vi "GOLPI Config Panel.vi"(8 "error in":errorcluster, 11 "session in":T2={"adc"={"niScope"={"channel cfg"=[], "sessions"=[], "multi cards"=FALSE, "channels"=0, "type"=enum."n/a", "memory [B/chn]"=0, "ext. clock [Hz]"=0.0, "samples count"=0, "use streaming"=FALSE, "proc setup"={"packet size [smpl]"=0, "current timeout [s]"=0.0, "blk2blk timeout [s]"=0.0, "event time"=timestamp(0 s since 1904-01-01), "temp sampl T [s]"=0.0, "data queue"=refnum, "stop notifier"=refnum, "proc ref"=refnum}, "sample width [B]"=0, "ranges [V]"=[], "trigger setup"={"coupling"=1, "level [V]"=0.0, "slope"=0, "mode"=enum."Immediate", "pre-trigger [%]"=0.0}, "fs [Hz]"=0.0, "bitres [bit]"=0, "clock source"=enum."VAL_NO_SOURCE"}, "3458A"={"channels"=[], "sync unit"={"VISA"="", "type"=enum."Picotest U6200A"}, "awg unit"={"type"=enum."Agilent 331xxA to 332xxA", "VISA"="", "enable 10MHz ref"=FALSE, "cmi ckd2"={"VISA"="", "clock source"=enum."Auto", "manual ref clk"=FALSE, "ref clock [Hz]"=0.0, "div mode"=enum."Set divisor directly"}, "cmi sync v3"={"VISA"="", "baud rate [bd/s]"=115200, "source"=enum."Auto", "hv range"=enum."1kV", "fsrc is fixed"=FALSE, "fsrc [Hz]"=10000000.0, "freq integ [s]"=1.0, "freq filter"=5, "trig level"=enum."TTL 5V", "chn1 mode"=enum."Source divider", "chn1 level"=enum."Positive 5V", "chn2 mode"=enum."Source divider", "chn2 level"=enum."Positive 5V", "chn2 div"=1, "chn3 mode"=enum."Chn 1 Active", "chn3 level"=enum."Positive 5V", "chn1 div entry"=enum."Calculate nearest divisor from measured fx", "chn1 dev limit [%]"=1.0, "chn1 check dev"=FALSE}, "trigger"={"source"=enum."Immediate", "slope"=enum."POS", "coupling"=enum."DC", "level [V]"=0.0, "hysteresis [V]"=0.0, "pre-trigger [%]"=0.0}, "HMF2500 cfg"={"Baud Rate"=9600, "Parity"=0, "Data Bits"=8, "Flow Control"=4}}, "sync mode"=enum."MASTER-SLAVE, MASTER clocked by TIMER", "streaming mode"=FALSE, "idn mode"=enum."Auto", "sampling mode"=enum."DCV", "sample memory [B]"=0, "proc setup"={"channel id"=0, "packet size [smpl]"=0, "current timeout [s]"=0.0, "blk2blk timeout [s]"=0.0, "event time"=timestamp(0 s since 1904-01-01), "stop notifier"=refnum, "data queues"=[], "proc refs"=[], "bus semaphore"=refnum}, "sample size [B]"=0, "sample count"=0, "aux data"={"channel id"=0, "valid?"=[], "gain [V]"=[], "timestamp [s]"=[], "Ts [s]"=0.0, "abs timestamp"=timestamp(0 s since 1904-01-01), "t [deg C]"=[], "multiplex timestamp [s]"=-1.0, "only multiplex?"=FALSE, "multiplex smpl offset"=0, "overflow?"=FALSE}, "ranges [V]"=[], "aperture [s]"=0.0, "LEVEL trigger"={"edge"=enum."POS", "level [V]"=0.0, "coupling"=enum."DC"}, "trigger mode"=enum."AUTO", "measure temp.?"=FALSE, "disp mesages"=[], "shared bus?"=FALSE, "disable display?"=FALSE, "aper mode"=enum."Manual", "aper rules"=[], "multiplex"={"cycles"=0, "delay [s]"=0.0, "enabled"=FALSE, "overhead [s]"=1.0, "tot smpls"=0, "sub-rec"=0, "overhead [%]"=0.0, "emulated"=FALSE}, "F8588 lpf"=enum."Off", "F8588 pll"=enum."Off", "F8588 couple"=enum."DC, auto", "fs"={"freq mode"=enum."fs or Ts", "fs [Hz]"=0.0, "fref [Hz]"=0.0, "mul"=0.0, "div"=0.0}, "fs mode"=enum."fs or Ts", "init timestamp"=timestamp(0 s since 1904-01-01), "last report timestamp"=timestamp(0 s since 1904-01-01)}, "dsdll"={"dsdll"={"dsdll path"=path "", "dsdll handle"=[], "output devices"=[], "capture devices"=[]}, "channels"=0, "device id"=0, "channel idns"=[], "proc setup"={"packet size [smpl]"=0, "current timeout [s]"=0.0, "blk2blk timeout [s]"=0.0, "event time"=timestamp(0 s since 1904-01-01), "data queue"=refnum, "stop notifier"=refnum, "proc ref"=refnum}, "samples count"=0, "fs [Hz]"=0.0}, "type"=enum."niScope", "channel idn str"=[], "aux instr idn str"=[], "modified?"=FALSE, "simadc"={"channels"=[], "range [V]"=0.0, "Ts step [s]"=0.0, "time [s]"=0.0, "fs [Hz]"=0.0, "count"=0, "smpl offset"=0, "set count"=0, "bit res"=0}, "force rst?"=FALSE, "exit mode"=enum."Immediate reset", "exit dly"=0.0, "exit tmr"=timestamp(0 s since 1904-01-01), "busy?"=FALSE, "accessed?"=FALSE, "multiplex"={"Type"=enum."Dummy", "gen com ssn"={"visa"="", "primary"=enum."None", "secondary"=enum."None", "channels"=[]}, "delay before [s]"=0.0, "delay post [s]"=0.0, "sequence"=[], "enabled"=FALSE, "ref timestamp [s]"=0.0, "idn string"="", "dev niScope"="", "niScope idx"=0, "QPMX ssn"={"visa"="", "switch mode"=enum."Switched by TWM", "sequence"=[], "timing delays"=[], "polarity"=enum."Positive", "ss delay (s)"=2.0, "internal timer (s)"=1.0, "Last loaded sequence file"=path "", "startup delay (s)"=2.0}, "VISA mux ssn"={"VISA"="", "paths"=[], "idn command"="", "serial cfg"={"Baud rate"=9600, "Data bits"=8, "Parity"=0, "Stop bits"=10, "Flow control"=0, "End Mode Read"=enum."None", "End Mode Write"=enum."None", "Term character"=0, "Term enable"=FALSE}}}, "keysight dso"={"VISA"="", "channels"=[], "bw limit [Hz]"=0.0, "resolution"=enum."Basic", "trig noise reject"=enum."Normal", "N"=0, "trigger config"={"trigger source"=enum."Immediate", "trigger slope"=enum."Negative", "level [V]"=0.0, "hysteresis [V]"=0.001, "pre-trig [%]"=50}, "fs [Hz]"=0.0, "timeout stop"=timestamp(0 s since 1904-01-01), "waiting for opc"=FALSE, "fetch offset [smpl]"=0, "abs timestamp"=timestamp(0 s since 1904-01-01), "ranges [V]"=[], "decimation"=1.0, "ext ref"=FALSE, "emulate aperture"=FALSE, "model"=enum."DSO91304"}, "cdaq"={"mclk [Hz]"=12800000.0, "ADC task"="", "mclk reference"="", "fs [Hz]"=50000.0, "queue adc cmd"=refnum, "queue adc data"=refnum, "adc proc ref"=refnum, "channels"=[], "last channels"=[], "timeout"=timestamp(0 s since 1904-01-01), "N"=1000, "mclk mode"=enum."Free running", "ext mclk source"=""}, "ignore overload"=FALSE, "ADS127L21"={"VISA"="", "chn list"=[], "record size"=0, "phys. channels"=0, "adc fifo size"=0, "channels"=[], "ext refclk?"=FALSE, "fs [Hz]"=0.0, "ext refclk [Hz]"=0.0, "meas refclk [Hz]"=0.0, "EXTOUT mode"=enum."ADCCLK", "EXTOUT polarity"=enum."NORM", "EXTOUT divisor"=0}}, "sequence"=[], "sequence setup"={"group setups"=[], "rec count"=0, "range mode"=enum."Keep defaults", "fs mode"=enum."Frequency", "rng even"=0.0, "rng odd"=0.0, "folder"=path "", "name base"="", "meas id"=0, "settle [s]"=0.0, "comment"="", "avg count"=0, "fs-abs-fr fr"=0.0, "fs-abs-fr fs"=0.0, "fs-div fr"=0.0, "fs-div div"=0.0, "fs-mn fr"=0.0, "fs-mn mul"=0.0, "fs-mn div"=0.0, "fs-rat fr"=0.0, "fs-rat rat"=0.0}, "golpi"=refnum, "processing setup"={"mode"=enum."Raw", "call after avgs?"=FALSE, "calculate?"=FALSE, "raw mode"={"command"="", "result mode"=enum."Display console output (only Octave)", "res variable"=""}, "QWTB"={"QWTB path"=path "", "alg filter path"="", "alg ids"=[], "alg parameters"=[], "parsed parameters"=[], "selected alg id"="", "selected unc mode"=enum."None", "qwtb mcc"=100, "qwtb timeout"=90, "qwtb covg"=95.0, "qwtb ofs"=0, "qwtb lim data"=0, "multicore"={"jobs folder"=path "", "cores"=0, "max jobs"=0, "mode"=enum."Singlecore"}, "unc once?"=FALSE, "qwtb tstemp"=enum."Enabled (default)", "octave reset"=FALSE, "exec mode"=enum."Single-core"}}, "corrections"={"transducers"={"channels"=[], "last path"=path "", "root path"=path ""}, "digitizer"={"last path"=path "", "channel paths"=[], "channel idns"=[], "correction name"="", "channel names"=[], "folders to copy"=[], "channel valid"=[], "correction path"=path "", "correction rel path"="", "rel folders to copy"=[], "root path"=path ""}}, "assist cfg"={"P"=0, "Q"=0, "rel shift"=0.0, "ref freq"=0.0, "min fs"=0.0, "max fs tol"=0.0, "min int"=0.0, "max int"=0.0, "max err"=0.0, "max timeout"=0.0}} {"corrections"."transducers"."channels"."Phase index" min=1 step=1; "adc"."ADS127L21"."channels"."Channel" min=1 max=8 step=1; "adc"."ADS127L21"."channels"."Range [Vpk]" items=["±1.65V", "±2V"]; "adc"."cdaq"."last channels"."Channel id" min=0 step=1; "adc"."cdaq"."channels"."Channel id" min=0 step=1; "adc"."keysight dso"."decimation" min=1.0; "adc"."keysight dso"."bw limit [Hz]" format="%#_6p"; "adc"."keysight dso"."channels"."Offset [V]" format="%#_6p"; "adc"."keysight dso"."channels"."Range [Vpk]" min=0.0 format="%#_6p"; "adc"."keysight dso"."channels"."Channel" min=1; "adc"."multiplex"."VISA mux ssn"."serial cfg"."Flow control" items=["None", "XON/XOFF", "CTS/RTS", "XON/XOFF + CTS/RTS", "DTR/DSR", "XON/XOFF + DTR/DSR"]; "adc"."multiplex"."VISA mux ssn"."serial cfg"."Stop bits" items=["1 bit"=10, "1.5 bits"=15, "2 bits"=20]; "adc"."multiplex"."VISA mux ssn"."serial cfg"."Parity" items=["None", "Odd", "Even", "Mark", "Space"]; "adc"."multiplex"."VISA mux ssn"."serial cfg"."Data bits" items=["5 bits"=5, "6 bits"=6, "7 bits"=7, "8 bits"=8]; "adc"."multiplex"."VISA mux ssn"."serial cfg"."Baud rate" items=["150 Bd"=150, "300 Bd"=300, "600 Bd"=600, "1200 Bd"=1200, "2400 Bd"=2400, "4800 Bd"=4800, "9600 Bd"=9600, "19.2 kBd"=19200, "38.4 kBd"=38400, "57.6 kBd"=57600, "115.2 kBd"=115200]; "adc"."multiplex"."QPMX ssn"."startup delay (s)" min=0.0 step=1.0; "adc"."multiplex"."QPMX ssn"."internal timer (s)" min=0.0 step=1.0; "adc"."multiplex"."QPMX ssn"."ss delay (s)" min=0.0 step=1.0; "adc"."multiplex"."QPMX ssn"."timing delays" min=1 max=255 step=1; "adc"."3458A"."awg unit"."HMF2500 cfg"."Flow Control" items=["None", "XON/XOFF", "RTS/CTS", "XON/XOFF & RTS/CTS", "DTR/DSR", "XON/XOFF & DTR/DSR"]; "adc"."3458A"."awg unit"."HMF2500 cfg"."Data Bits" items=["7"=7, "8"=8]; "adc"."3458A"."awg unit"."HMF2500 cfg"."Parity" items=["None", "Odd", "Even", "Mark", "Space"]; "adc"."3458A"."awg unit"."HMF2500 cfg"."Baud Rate" items=["300"=300, "600"=600, "1200"=1200, "2400"=2400, "4800"=4800, "9600"=9600, "19200"=19200]; "adc"."3458A"."awg unit"."cmi sync v3"."chn2 div" min=1 max=100000000 step=1; "adc"."3458A"."awg unit"."cmi sync v3"."fsrc [Hz]" format="%_8p"; "adc"."3458A"."channels"."Range [Vpk]" min=0.0; "adc"."niScope"."trigger setup"."pre-trigger [%]" format="%.2f"; "adc"."niScope"."trigger setup"."level [V]" format="%.2f"; "adc"."niScope"."trigger setup"."coupling" items=["AC"=0, "DC"=1, "HF Reject"=3, "LF Reject"=4, "AC Plus HF Reject"=1001]; "adc"."niScope"."channel cfg"."Range [Vpk]" min=0.0; "adc"."niScope"."channel cfg"."Channel" min=0}) -> (0 "error out":errorcluster, 3 "session out":T2={"adc"={"niScope"={"channel cfg"=[], "sessions"=[], "multi cards"=FALSE, "channels"=0, "type"=enum."n/a", "memory [B/chn]"=0, "ext. clock [Hz]"=0.0, "samples count"=0, "use streaming"=FALSE, "proc setup"={"packet size [smpl]"=0, "current timeout [s]"=0.0, "blk2blk timeout [s]"=0.0, "event time"=timestamp(0 s since 1904-01-01), "temp sampl T [s]"=0.0, "data queue"=refnum, "stop notifier"=refnum, "proc ref"=refnum}, "sample width [B]"=0, "ranges [V]"=[], "trigger setup"={"coupling"=1, "level [V]"=0.0, "slope"=0, "mode"=enum."Immediate", "pre-trigger [%]"=0.0}, "fs [Hz]"=0.0, "bitres [bit]"=0, "clock source"=enum."VAL_NO_SOURCE"}, "3458A"={"channels"=[], "sync unit"={"VISA"="", "type"=enum."Picotest U6200A"}, "awg unit"={"type"=enum."Agilent 331xxA to 332xxA", "VISA"="", "enable 10MHz ref"=FALSE, "cmi ckd2"={"VISA"="", "clock source"=enum."Auto", "manual ref clk"=FALSE, "ref clock [Hz]"=0.0, "div mode"=enum."Set divisor directly"}, "cmi sync v3"={"VISA"="", "baud rate [bd/s]"=115200, "source"=enum."Auto", "hv range"=enum."1kV", "fsrc is fixed"=FALSE, "fsrc [Hz]"=10000000.0, "freq integ [s]"=1.0, "freq filter"=5, "trig level"=enum."TTL 5V", "chn1 mode"=enum."Source divider", "chn1 level"=enum."Positive 5V", "chn2 mode"=enum."Source divider", "chn2 level"=enum."Positive 5V", "chn2 div"=1, "chn3 mode"=enum."Chn 1 Active", "chn3 level"=enum."Positive 5V", "chn1 div entry"=enum."Calculate nearest divisor from measured fx", "chn1 dev limit [%]"=1.0, "chn1 check dev"=FALSE}, "trigger"={"source"=enum."Immediate", "slope"=enum."POS", "coupling"=enum."DC", "level [V]"=0.0, "hysteresis [V]"=0.0, "pre-trigger [%]"=0.0}, "HMF2500 cfg"={"Baud Rate"=9600, "Parity"=0, "Data Bits"=8, "Flow Control"=4}}, "sync mode"=enum."MASTER-SLAVE, MASTER clocked by TIMER", "streaming mode"=FALSE, "idn mode"=enum."Auto", "sampling mode"=enum."DCV", "sample memory [B]"=0, "proc setup"={"channel id"=0, "packet size [smpl]"=0, "current timeout [s]"=0.0, "blk2blk timeout [s]"=0.0, "event time"=timestamp(0 s since 1904-01-01), "stop notifier"=refnum, "data queues"=[], "proc refs"=[], "bus semaphore"=refnum}, "sample size [B]"=0, "sample count"=0, "aux data"={"channel id"=0, "valid?"=[], "gain [V]"=[], "timestamp [s]"=[], "Ts [s]"=0.0, "abs timestamp"=timestamp(0 s since 1904-01-01), "t [deg C]"=[], "multiplex timestamp [s]"=-1.0, "only multiplex?"=FALSE, "multiplex smpl offset"=0, "overflow?"=FALSE}, "ranges [V]"=[], "aperture [s]"=0.0, "LEVEL trigger"={"edge"=enum."POS", "level [V]"=0.0, "coupling"=enum."DC"}, "trigger mode"=enum."AUTO", "measure temp.?"=FALSE, "disp mesages"=[], "shared bus?"=FALSE, "disable display?"=FALSE, "aper mode"=enum."Manual", "aper rules"=[], "multiplex"={"cycles"=0, "delay [s]"=0.0, "enabled"=FALSE, "overhead [s]"=1.0, "tot smpls"=0, "sub-rec"=0, "overhead [%]"=0.0, "emulated"=FALSE}, "F8588 lpf"=enum."Off", "F8588 pll"=enum."Off", "F8588 couple"=enum."DC, auto", "fs"={"freq mode"=enum."fs or Ts", "fs [Hz]"=0.0, "fref [Hz]"=0.0, "mul"=0.0, "div"=0.0}, "fs mode"=enum."fs or Ts", "init timestamp"=timestamp(0 s since 1904-01-01), "last report timestamp"=timestamp(0 s since 1904-01-01)}, "dsdll"={"dsdll"={"dsdll path"=path "", "dsdll handle"=[], "output devices"=[], "capture devices"=[]}, "channels"=0, "device id"=0, "channel idns"=[], "proc setup"={"packet size [smpl]"=0, "current timeout [s]"=0.0, "blk2blk timeout [s]"=0.0, "event time"=timestamp(0 s since 1904-01-01), "data queue"=refnum, "stop notifier"=refnum, "proc ref"=refnum}, "samples count"=0, "fs [Hz]"=0.0}, "type"=enum."niScope", "channel idn str"=[], "aux instr idn str"=[], "modified?"=FALSE, "simadc"={"channels"=[], "range [V]"=0.0, "Ts step [s]"=0.0, "time [s]"=0.0, "fs [Hz]"=0.0, "count"=0, "smpl offset"=0, "set count"=0, "bit res"=0}, "force rst?"=FALSE, "exit mode"=enum."Immediate reset", "exit dly"=0.0, "exit tmr"=timestamp(0 s since 1904-01-01), "busy?"=FALSE, "accessed?"=FALSE, "multiplex"={"Type"=enum."Dummy", "gen com ssn"={"visa"="", "primary"=enum."None", "secondary"=enum."None", "channels"=[]}, "delay before [s]"=0.0, "delay post [s]"=0.0, "sequence"=[], "enabled"=FALSE, "ref timestamp [s]"=0.0, "idn string"="", "dev niScope"="", "niScope idx"=0, "QPMX ssn"={"visa"="", "switch mode"=enum."Switched by TWM", "sequence"=[], "timing delays"=[], "polarity"=enum."Positive", "ss delay (s)"=2.0, "internal timer (s)"=1.0, "Last loaded sequence file"=path "", "startup delay (s)"=2.0}, "VISA mux ssn"={"VISA"="", "paths"=[], "idn command"="", "serial cfg"={"Baud rate"=9600, "Data bits"=8, "Parity"=0, "Stop bits"=10, "Flow control"=0, "End Mode Read"=enum."None", "End Mode Write"=enum."None", "Term character"=0, "Term enable"=FALSE}}}, "keysight dso"={"VISA"="", "channels"=[], "bw limit [Hz]"=0.0, "resolution"=enum."Basic", "trig noise reject"=enum."Normal", "N"=0, "trigger config"={"trigger source"=enum."Immediate", "trigger slope"=enum."Negative", "level [V]"=0.0, "hysteresis [V]"=0.001, "pre-trig [%]"=50}, "fs [Hz]"=0.0, "timeout stop"=timestamp(0 s since 1904-01-01), "waiting for opc"=FALSE, "fetch offset [smpl]"=0, "abs timestamp"=timestamp(0 s since 1904-01-01), "ranges [V]"=[], "decimation"=1.0, "ext ref"=FALSE, "emulate aperture"=FALSE, "model"=enum."DSO91304"}, "cdaq"={"mclk [Hz]"=12800000.0, "ADC task"="", "mclk reference"="", "fs [Hz]"=50000.0, "queue adc cmd"=refnum, "queue adc data"=refnum, "adc proc ref"=refnum, "channels"=[], "last channels"=[], "timeout"=timestamp(0 s since 1904-01-01), "N"=1000, "mclk mode"=enum."Free running", "ext mclk source"=""}, "ignore overload"=FALSE, "ADS127L21"={"VISA"="", "chn list"=[], "record size"=0, "phys. channels"=0, "adc fifo size"=0, "channels"=[], "ext refclk?"=FALSE, "fs [Hz]"=0.0, "ext refclk [Hz]"=0.0, "meas refclk [Hz]"=0.0, "EXTOUT mode"=enum."ADCCLK", "EXTOUT polarity"=enum."NORM", "EXTOUT divisor"=0}}, "sequence"=[], "sequence setup"={"group setups"=[], "rec count"=0, "range mode"=enum."Keep defaults", "fs mode"=enum."Frequency", "rng even"=0.0, "rng odd"=0.0, "folder"=path "", "name base"="", "meas id"=0, "settle [s]"=0.0, "comment"="", "avg count"=0, "fs-abs-fr fr"=0.0, "fs-abs-fr fs"=0.0, "fs-div fr"=0.0, "fs-div div"=0.0, "fs-mn fr"=0.0, "fs-mn mul"=0.0, "fs-mn div"=0.0, "fs-rat fr"=0.0, "fs-rat rat"=0.0}, "golpi"=refnum, "processing setup"={"mode"=enum."Raw", "call after avgs?"=FALSE, "calculate?"=FALSE, "raw mode"={"command"="", "result mode"=enum."Display console output (only Octave)", "res variable"=""}, "QWTB"={"QWTB path"=path "", "alg filter path"="", "alg ids"=[], "alg parameters"=[], "parsed parameters"=[], "selected alg id"="", "selected unc mode"=enum."None", "qwtb mcc"=100, "qwtb timeout"=90, "qwtb covg"=95.0, "qwtb ofs"=0, "qwtb lim data"=0, "multicore"={"jobs folder"=path "", "cores"=0, "max jobs"=0, "mode"=enum."Singlecore"}, "unc once?"=FALSE, "qwtb tstemp"=enum."Enabled (default)", "octave reset"=FALSE, "exec mode"=enum."Single-core"}}, "corrections"={"transducers"={"channels"=[], "last path"=path "", "root path"=path ""}, "digitizer"={"last path"=path "", "channel paths"=[], "channel idns"=[], "correction name"="", "channel names"=[], "folders to copy"=[], "channel valid"=[], "correction path"=path "", "correction rel path"="", "rel folders to copy"=[], "root path"=path ""}}, "assist cfg"={"P"=0, "Q"=0, "rel shift"=0.0, "ref freq"=0.0, "min fs"=0.0, "max fs tol"=0.0, "min int"=0.0, "max int"=0.0, "max err"=0.0, "max timeout"=0.0}} {"corrections"."transducers"."channels"."Phase index" min=1 step=1; "adc"."ADS127L21"."channels"."Channel" min=1 max=8 step=1; "adc"."ADS127L21"."channels"."Range [Vpk]" items=["±1.65V", "±2V"]; "adc"."cdaq"."last channels"."Channel id" min=0 step=1; "adc"."cdaq"."channels"."Channel id" min=0 step=1; "adc"."keysight dso"."decimation" min=1.0; "adc"."keysight dso"."bw limit [Hz]" format="%#_6p"; "adc"."keysight dso"."channels"."Offset [V]" format="%#_6p"; "adc"."keysight dso"."channels"."Range [Vpk]" min=0.0 format="%#_6p"; "adc"."keysight dso"."channels"."Channel" min=1; "adc"."multiplex"."VISA mux ssn"."serial cfg"."Flow control" items=["None", "XON/XOFF", "CTS/RTS", "XON/XOFF + CTS/RTS", "DTR/DSR", "XON/XOFF + DTR/DSR"]; "adc"."multiplex"."VISA mux ssn"."serial cfg"."Stop bits" items=["1 bit"=10, "1.5 bits"=15, "2 bits"=20]; "adc"."multiplex"."VISA mux ssn"."serial cfg"."Parity" items=["None", "Odd", "Even", "Mark", "Space"]; "adc"."multiplex"."VISA mux ssn"."serial cfg"."Data bits" items=["5 bits"=5, "6 bits"=6, "7 bits"=7, "8 bits"=8]; "adc"."multiplex"."VISA mux ssn"."serial cfg"."Baud rate" items=["150 Bd"=150, "300 Bd"=300, "600 Bd"=600, "1200 Bd"=1200, "2400 Bd"=2400, "4800 Bd"=4800, "9600 Bd"=9600, "19.2 kBd"=19200, "38.4 kBd"=38400, "57.6 kBd"=57600, "115.2 kBd"=115200]; "adc"."multiplex"."QPMX ssn"."startup delay (s)" min=0.0 step=1.0; "adc"."multiplex"."QPMX ssn"."internal timer (s)" min=0.0 step=1.0; "adc"."multiplex"."QPMX ssn"."ss delay (s)" min=0.0 step=1.0; "adc"."multiplex"."QPMX ssn"."timing delays" min=1 max=255 step=1; "adc"."3458A"."awg unit"."HMF2500 cfg"."Flow Control" items=["None", "XON/XOFF", "RTS/CTS", "XON/XOFF & RTS/CTS", "DTR/DSR", "XON/XOFF & DTR/DSR"]; "adc"."3458A"."awg unit"."HMF2500 cfg"."Data Bits" items=["7"=7, "8"=8]; "adc"."3458A"."awg unit"."HMF2500 cfg"."Parity" items=["None", "Odd", "Even", "Mark", "Space"]; "adc"."3458A"."awg unit"."HMF2500 cfg"."Baud Rate" items=["300"=300, "600"=600, "1200"=1200, "2400"=2400, "4800"=4800, "9600"=9600, "19200"=19200]; "adc"."3458A"."awg unit"."cmi sync v3"."chn2 div" min=1 max=100000000 step=1; "adc"."3458A"."awg unit"."cmi sync v3"."fsrc [Hz]" format="%_8p"; "adc"."3458A"."channels"."Range [Vpk]" min=0.0; "adc"."niScope"."trigger setup"."pre-trigger [%]" format="%.2f"; "adc"."niScope"."trigger setup"."level [V]" format="%.2f"; "adc"."niScope"."trigger setup"."coupling" items=["AC"=0, "DC"=1, "HF Reject"=3, "LF Reject"=4, "AC Plus HF Reject"=1001]; "adc"."niScope"."channel cfg"."Range [Vpk]" min=0.0; "adc"."niScope"."channel cfg"."Channel" min=0})   [LabVIEW 2020]
doc: "This is panel for configuration of Octave/Matlab interface."
uses:
  measure/Meas Session.ctl
  adc/ADC Session.ctl
  drivers/niScope/niScope Session.ctl
  drivers/niScope/niScope Virtual Channel Config.ctl
  drivers/niScope/niScope Virtual Channel Mode.ctl
  drivers/niScope/niScope Virtual Channel Input Z.ctl
  drivers/niScope/niScope Virtual Channel Coupling.ctl
  drivers/niScope/niScope Type.ctl
  drivers/niScope/niScope Digitizing Process Options.ctl
  drivers/niScope/niScope Data Packet.ctl
  drivers/niScope/niScope Trigger Setup.ctl
  <instrlib>/niScope/Controls/niScope trigger coupling.ctl
  <instrlib>/niScope/Controls/niScope trigger slope.ctl
  drivers/niScope/niScope Reference Clock.ctl
  drivers/DMM/3458A Digitizer Session.ctl
  drivers/DMM/3458A Virtual Channel Config.ctl
  drivers/Counter/Counter Session.ctl
  drivers/Counter/Counter Type.ctl
  drivers/AWG/AWG Session.ctl
  drivers/AWG/AWG Type.ctl
  drivers/AWG/CMI Clock Divider v2/CMI ckd2 Session.ctl
  drivers/AWG/CMI Clock Divider v2/CMI ckd2 Source Mode.ctl
  drivers/AWG/CMI Clock Divider v2/CMI ckd2 Divisor Mode.ctl
  drivers/AWG/CMI Sync V3/CMI Sync V3 session.ctl
  drivers/AWG/CMI Sync V3/Configure/CMI Sync V3 Reference Clock Source.ctl
  drivers/AWG/CMI Sync V3/Configure/CMI Sync V3 HV input Range.ctl
  drivers/AWG/CMI Sync V3/Configure/CMI Sync V3 Trigger Input Level.ctl
  drivers/AWG/CMI Sync V3/Configure/CMI Sync V3 Channel 1 Mode.ctl
  drivers/AWG/CMI Sync V3/Configure/CMI Sync V3 Channel Output Levels.ctl
  drivers/AWG/CMI Sync V3/Configure/CMI Sync V3 Channel 2 Mode.ctl
  drivers/AWG/CMI Sync V3/Configure/CMI Sync V3 Channel 3 Mode.ctl
  drivers/AWG/CMI Sync V3/Configure/CMI Sync V3 Channel 1 Divisor Entry Mode.ctl
  adc/ADC Trig Config.ctl
  adc/ADC Trig Mode Source.ctl
  adc/ADC Trig Slope.ctl
  adc/ADC Trig Coupling.ctl
  drivers/AWG/RaS HMF2500/HMF2500 Config.ctl
  drivers/DMM/3458A Sync Mode.ctl
  drivers/DMM/3458A Idn Mode.ctl
  drivers/DMM/3458A Digitizing Low Levels/Configure/Sampling Mode.ctl
  drivers/DMM/3458A Digitizing Process Options.ctl
  drivers/DMM/3458A Data Packet.ctl
  drivers/DMM/3458A Aux Record Data.ctl
  drivers/DMM/3458A Digitizing Low Levels/Configure/Level Setup.ctl
  drivers/DMM/3458A Digitizing Low Levels/Configure/First Sample Trigger.ctl
  drivers/DMM/3458A Aperture Selection Mode.ctl
  drivers/DMM/3458A Multiplexing Config.ctl
  drivers/Fluke 8588A/F8588A Low Pass Filter.ctl
  drivers/Fluke 8588A/F8588A Phase Lock.ctl
  drivers/Fluke 8588A/F8588A Coupling.ctl
  drivers/DMM/3458A Sampling Rate.ctl
  drivers/AWG/AWG Clock Setup Mode.ctl
  drivers/DMM/3458A Sample Rate Mode.ctl
  drivers/dsdll/DSDLL Session.ctl
  drivers/dsdll/dsdll/dsdll_instance.ctl
  drivers/dsdll/dsdll/dsdll_device_record.ctl
  drivers/dsdll/DSDLL Process Config.ctl
  drivers/dsdll/DSDLL Data Packet.ctl
  adc/ADC Type.ctl
  drivers/simulated_adc/SimAdc Config.ctl
  drivers/simulated_adc/SimAdc Channel Cfg.ctl
  adc/ADC On Close Action.ctl
  adc/Multiplexer/MPX Session.ctl
  adc/Multiplexer/MPX Type.ctl
  drivers/Multiplexers/Generic COM/GCOMM Session.ctl
  drivers/Multiplexers/Generic COM/GCOMM Signal.ctl
  drivers/Multiplexers/Generic COM/GCOMM Virtual Channel.ctl
  drivers/Multiplexers/Generic COM/GCOMM Logic State.ctl
  drivers/Multiplexers/Generic COM/QPMX Session.ctl
  drivers/Multiplexers/QPMX/QPMX switch mode.ctl
  drivers/Multiplexers/QPMX/QPMX polarity.ctl
  drivers/Multiplexers/Generic VISA commands/GVISA Mux Session.ctl
  drivers/Multiplexers/Generic VISA commands/GVISA Mux Path Entry.ctl
  drivers/Multiplexers/Generic VISA commands/met_serial_setup.ctl
  drivers/Agilent DSO 90000/Virtual Digitizer/KeDSO session.ctl
  drivers/Agilent DSO 90000/Virtual Digitizer/KeDSO Virtual Channel.ctl
  drivers/Agilent DSO 90000/Virtual Digitizer/KeDSO High Resolution Mode.ctl
  drivers/Agilent DSO 90000/Virtual Digitizer/KeDSO Trigger Setup.ctl
  drivers/Agilent DSO 90000/Virtual Digitizer/KeDSO Trigger Source.ctl
  drivers/Agilent DSO 90000/Public/Utility/DSO type.ctl
  drivers/cdaq/cDAQ Session.ctl
  drivers/cdaq/low_level_old/cdaq_anal_adc_command.ctl
  drivers/cdaq/low_level_old/cdaq_anal_adc_data.ctl
  drivers/cdaq/cDAQ Virtual Channel.ctl
  drivers/cdaq/cDAQ Master Clock Mode.ctl
  drivers/CMI_ADS127L21/CMI ADS127L21 - Session.ctl
  drivers/CMI_ADS127L21/CMI ADS127L21 - Record Channel.ctl
  drivers/CMI_ADS127L21/CMI ADS127L21 - Input Range.ctl
  drivers/CMI_ADS127L21/CMI ADS127L21 - Input Mode.ctl
  drivers/CMI_ADS127L21/CMI ADS127L21 - Input Impedance.ctl
  drivers/CMI_ADS127L21/CMI ADS127L21 - EXTOUT Mode.ctl
  drivers/CMI_ADS127L21/CMI ADS127L21 - EXTOUT Polarity.ctl
  measure/Meas Sequence Item.ctl
  measure/Meas Sampling Configuration.ctl
  measure/processing/QWTB/Meas Proc QWTB Algorithm Parameter Data.ctl
  measure/Meas Sequence Configuration.ctl
  measure/Meas Range Mode.ctl
  measure/Meas Sampling Rate Mode.ctl
  golpi_session_ref.ctl
  golpi_session.ctl
  GOLPI reference Type Def.ctl
  Pipe Handle.ctl
  measure/processing/Meas Process Config.ctl
  measure/processing/Meas Process Mode.ctl
  measure/processing/Meas Process Raw Config.ctl
  measure/processing/Meas Process Raw Result Mode.ctl
  measure/processing/QWTB/Meas Proc QWTB Setup.ctl
  measure/processing/QWTB/Meas Proc QWTB Uncertainty Mode.ctl
  measure/processing/QWTB/Meas Proc QWTB Multicore Setup.ctl
  measure/processing/QWTB/Meas Proc QWTB Multicore Type.ctl
  measure/processing/Meas Process Time Stamp Mode.ctl
  measure/processing/QWTB/Meas Proc QWTB Exec Mode.ctl
  measure/Corrections/Corr Setup.ctl
  measure/Corrections/Corr Tranducer Item.ctl
  measure/Corrections/Corr Digitizers.ctl
  measure/Assist/Assist Panel Setup.ctl
  varilib/SGUI Assign References Mode.ctl
  varilib/SGUI Assign Multiple Strings With Tags By Label.vi
  varilib/varilib.lvlib
  GOLPI library.lvlib
  GOLPI Multi Process.lvlib
  drivers/niScope/niScope Virtual Digitizer.lvlib
  drivers/DMM/3458A Virtual Digitizer.lvlib
  drivers/Counter/Counter.lvlib
  drivers/AWG/AWG.lvlib
  drivers/DMM/3458A Digitizing Low Levels/3458A Digitizing Low Levels.lvlib
  drivers/dsdll/DSDLL Virtual Digitizer.lvlib
  drivers/dsdll/dsdll/dsdll.lvlib
  LV Process library.lvlib
  drivers/AWG/CMI Sync V3/CMI Sync Unit V3.lvlib
  drivers/Agilent DSO 90000/Agilent 90000 Series.lvlib
panel:
  in  "help":bool caption="Help"
  in  "btn default":bool caption="Default"
  out "golpi":T1
  in  "tc qwtb":enum32{"Page 1", "Page 2"}(tab) caption="QWTB related"
  in  "qwtb filter":string caption="Relative path to the QWTB algorithms filter (list of supported algorithms)"
  out "qwtb status":bool caption="QWTB status"
  in  "btn test qwtb":bool caption="Test QWTB"
  in  "qwtb path":path caption="QWTB toolbox root folder path (optional)"
  out "qwtb stat str":string caption="Status"
  in  "btn stop":bool caption="Stop GOLPI"
  in  "tc golpi stat":enum32{"Page 1", "Page 2"}(tab) caption="Status frame"
  out "status":bool
  out "ver":string caption="GNU Octave / Matlab version"
  out "golpi stat":bool caption="GNU Octave or communication with Matlab running?"
  in  "btn test":bool caption="Restart"
  in  "btn ok":bool caption="OK"
  in  "tc main":enum32{"Page 1", "Page 2"}(tab) caption="Frame settings"
  in  "btn edit exit":bool caption="Edit at_exit.m"
  in  "btn edit startup":bool caption="Edit at_startup.m"
  in  "btn matlab":bool caption="Enable Matlab Script mode"
  in  "btn clr cache":bool caption="Always clear function cache (slower)"
  in  "btn bitstream":bool caption="Use bitstream mode"
  in  "btn console":bool caption="Show console window"
  in  "start timeout [ms]":u32=30000 caption="Startup timeout [ms]"
  in  "octave path":path=path "C:/Octave/Octave_3.6.4/bin" caption="GNU Octave binary path (folder or full path)"
  in  "btn pkg ass":bool caption="Package Assist"
  # "Note: Restart GOLPI to apply changes!"
  # "ADC:"
  # "ADC:"
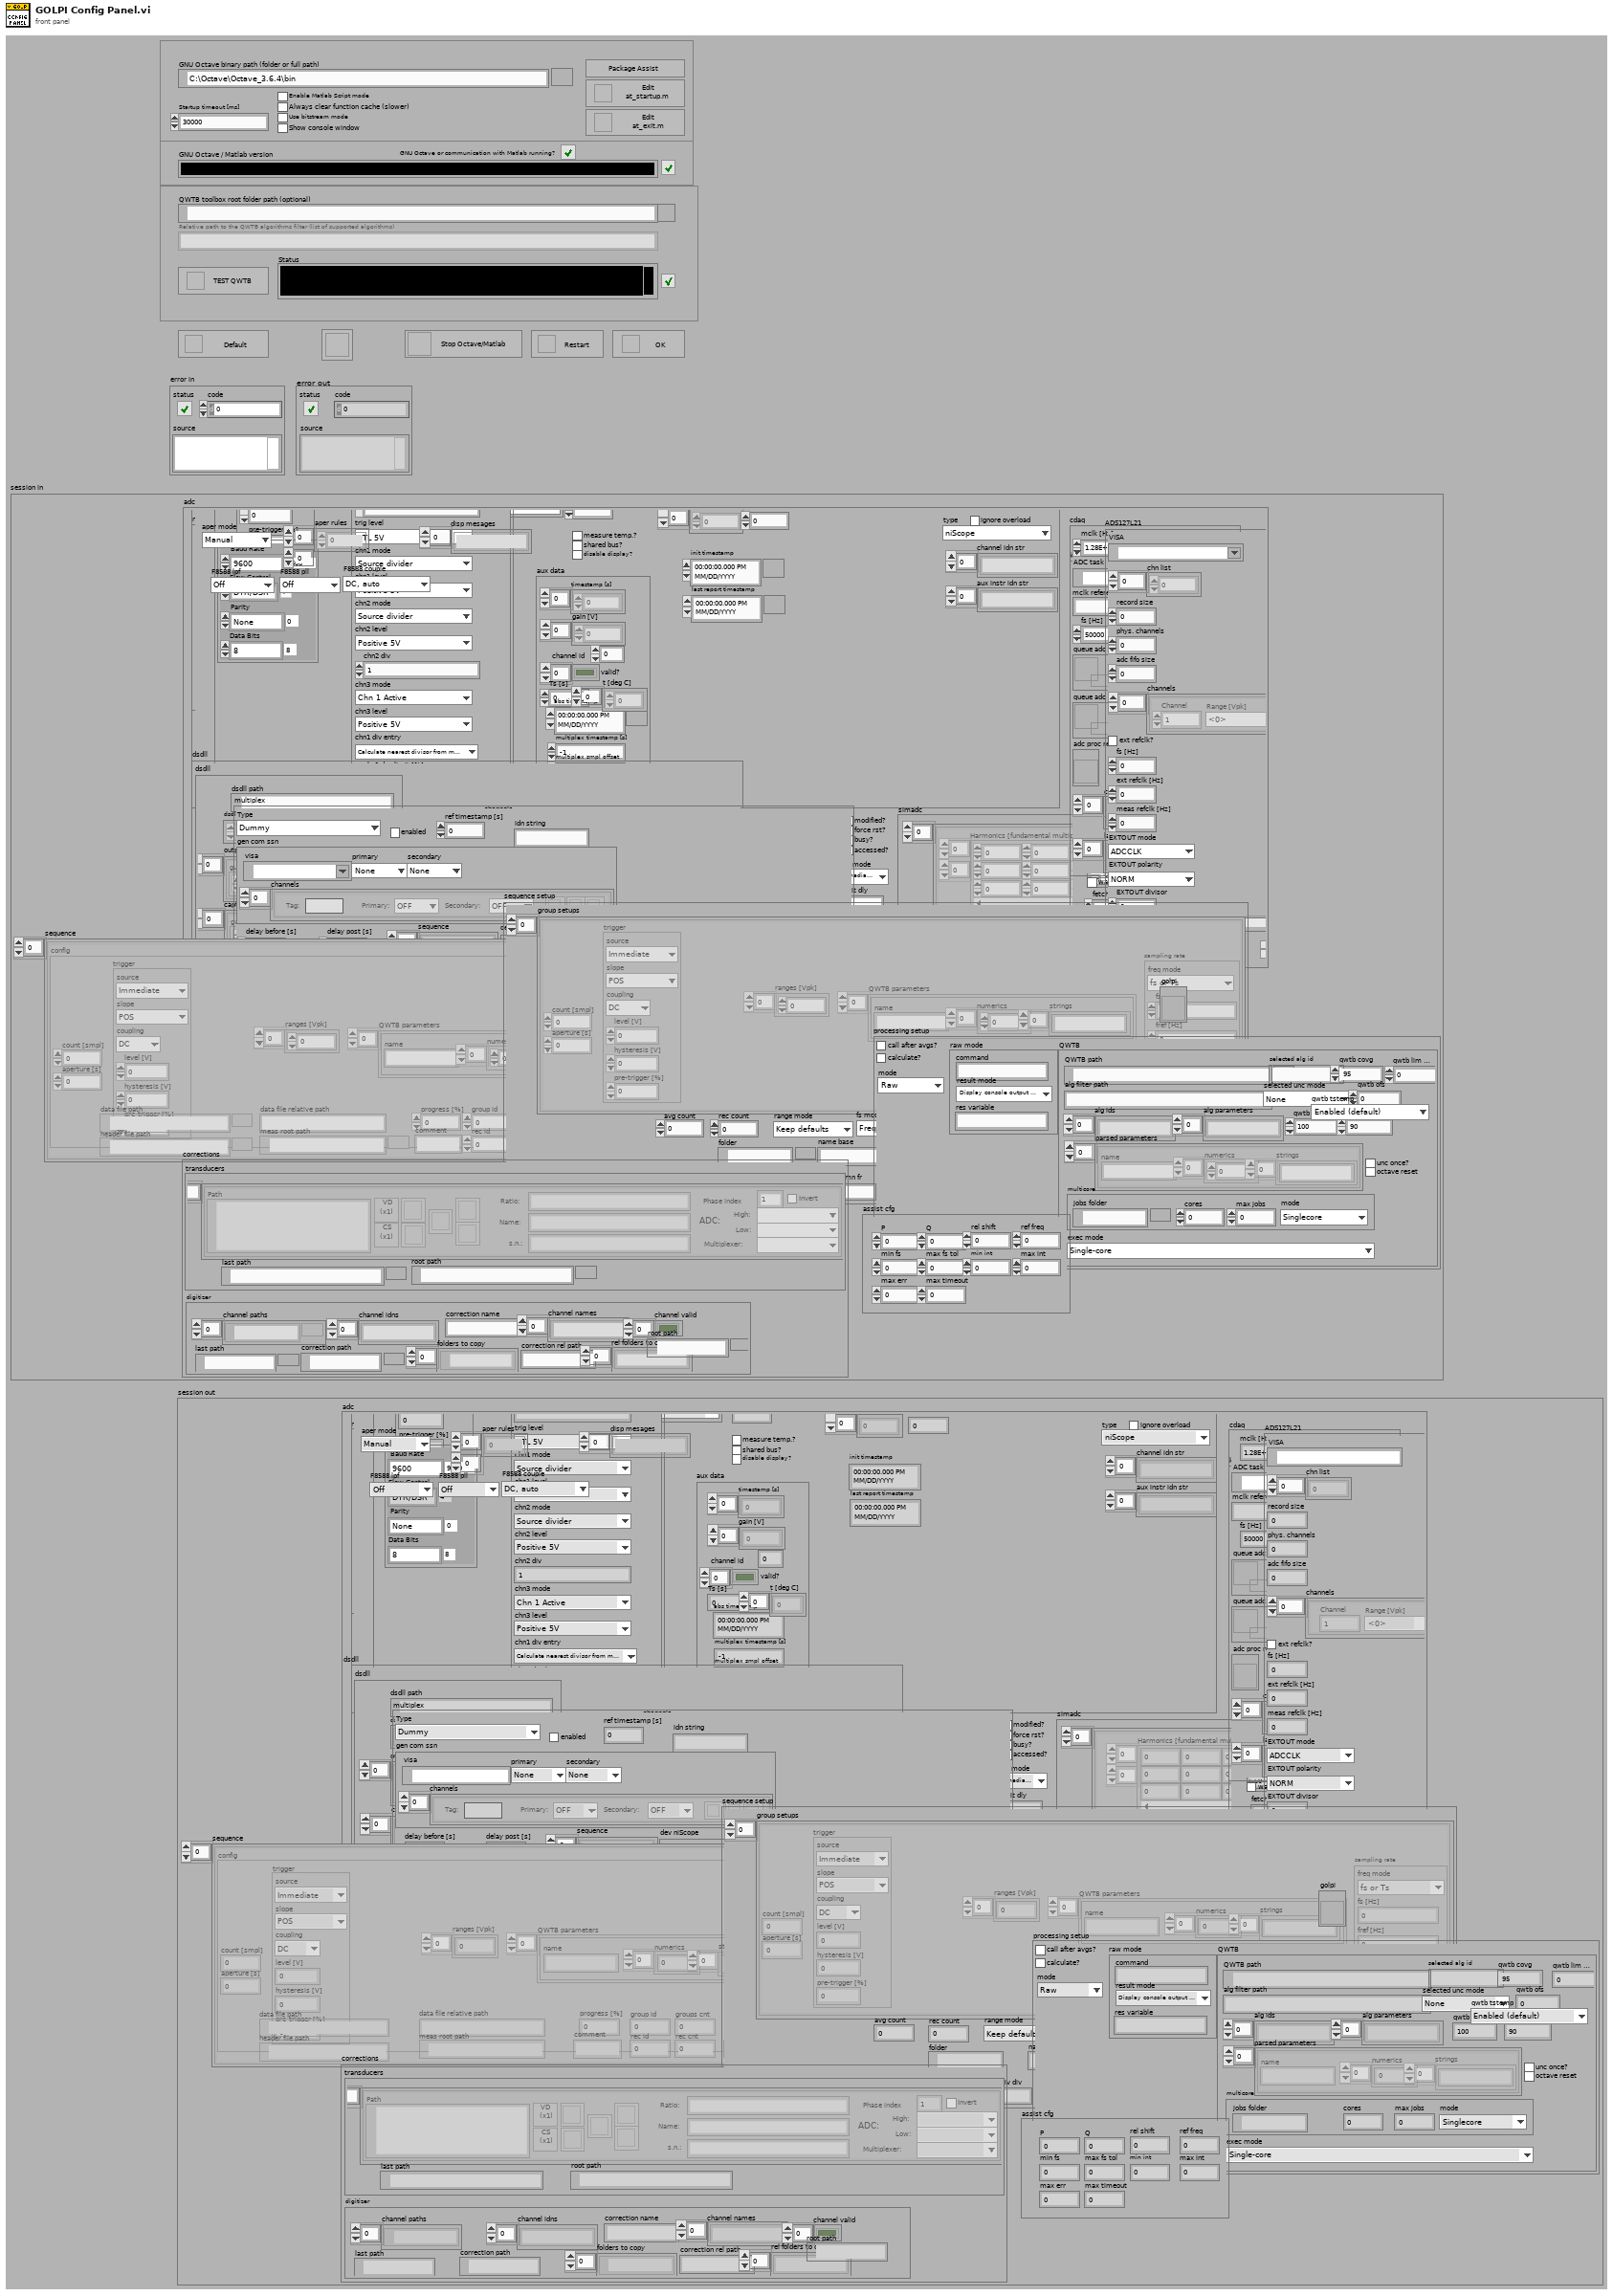
[diagram p1: front panel]
types:
  T1 = typedef "GOLPI Multi Process.lvlib/golpi_session_ref.ctl" = refnum<vi>
  T2 = typedef "Meas Session.ctl" = cluster{"adc":T3, "sequence":T90[], "sequence setup":T93, "golpi":T1, "processing setup":T96, "corrections":T106, "assist cfg":T109}
  T3 = typedef "ADC Session.ctl" = cluster{"niScope":T4, "3458A":T15, "dsdll":T54, "type":T58, "channel idn str":string[], "aux instr idn str":string[], "modified?":bool, "simadc":T59, "force rst?":bool, "exit mode":T61, "exit dly":dbl, "exit tmr":timestamp, "busy?":bool, "accessed?":bool, "multiplex":T62, "keysight dso":T74, "cdaq":T80, "ignore overload":bool, "ADS127L21":T83}
  T4 = typedef "niScope Virtual Digitizer.lvlib/niScope Session.ctl" = cluster{"channel cfg":T5[], "sessions":refnum<k20>[], "multi cards":bool, "channels":i32, "type":T9, "memory [B/chn]":i32, "ext. clock [Hz]":dbl, "samples count":i64, "use streaming":bool, "proc setup":T10, "sample width [B]":i32, "ranges [V]":dbl[], "trigger setup":T11, "fs [Hz]":dbl, "bitres [bit]":i32, "clock source":T14}
  T5 = typedef "niScope Virtual Digitizer.lvlib/niScope Virtual Channel Config.ctl" = cluster{"Address":refnum<k15>, "Channel":i32, "Mode":T6, "Input Z":T7, "Coupling":T8, "Range [Vpk]":dbl, "btn clr":bool, "btn up":bool, "btn down":bool}
  T6 = typedef "niScope Virtual Digitizer.lvlib/niScope Virtual Channel Mode.ctl" = enum16{"Single ended", "Unbal. differential", "Differential"}
  T7 = typedef "niScope Virtual Digitizer.lvlib/niScope Virtual Channel Input Z.ctl" = enum16{"1 MOhm", "50 Ohm"}
  T8 = typedef "niScope Virtual Digitizer.lvlib/niScope Virtual Channel Coupling.ctl" = enum16{"AC", "DC", "GND"}
  T9 = typedef "niScope Virtual Digitizer.lvlib/niScope Type.ctl" = enum16{"n/a", "5922"}
  T10 = typedef "niScope Virtual Digitizer.lvlib/niScope Digitizing Process Options.ctl" = cluster{"packet size [smpl]":i64, "current timeout [s]":dbl, "blk2blk timeout [s]":dbl, "event time":timestamp, "temp sampl T [s]":dbl, "data queue":refnum<queue>, "stop notifier":refnum<notifier>, "proc ref":refnum<vi>}
  T11 = typedef "niScope Virtual Digitizer.lvlib/niScope Trigger Setup.ctl" = cluster{"coupling":T12, "level [V]":dbl, "slope":T13, "mode":enum16{"Immediate", "External", "Level"}, "pre-trigger [%]":dbl}
  T12 = typedef "niScope trigger coupling.ctl" = u16
  T13 = typedef "niScope trigger slope.ctl" = i32
  T14 = typedef "niScope Virtual Digitizer.lvlib/niScope Reference Clock.ctl" = enum16{"VAL_NO_SOURCE", "VAL_CLK_IN", "VAL_PXI_CLOCK", "VAL_EXTERNAL"}
  T15 = typedef "3458A Virtual Digitizer.lvlib/3458A Digitizer Session.ctl" = cluster{"channels":T16[], "sync unit":T17, "awg unit":T19, "sync mode":T38, "streaming mode":bool, "idn mode":T39, "sampling mode":T40, "sample memory [B]":i32, "proc setup":T41, "sample size [B]":i32, "sample count":i32, "aux data":T43, "ranges [V]":dbl[], "aperture [s]":dbl, "LEVEL trigger":T44, "trigger mode":T45, "measure temp.?":bool, "disp mesages":string[], "shared bus?":bool, "disable display?":bool, "aper mode":T46, "aper rules":dbl[][], "multiplex":T47, "F8588 lpf":T48, "F8588 pll":T49, "F8588 couple":T50, "fs":T51, "fs mode":T53, "init timestamp":timestamp, "last report timestamp":timestamp}
  T16 = typedef "3458A Virtual Digitizer.lvlib/3458A Virtual Channel Config.ctl" = cluster{"VISA":refnum<visa-resource-name>, "Range [Vpk]":dbl, "btn clr":bool, "btn up":bool, "btn down":bool, "F8588":bool, "F8588 guard":bool}
  T17 = typedef "Counter.lvlib/Counter Session.ctl" = cluster{"VISA":refnum<visa-resource-name>, "type":T18}
  T18 = typedef "Counter.lvlib/Counter Type.ctl" = enum16{"Picotest U6200A", "dummy"}
  T19 = typedef "AWG.lvlib/AWG Session.ctl" = cluster{"type":T20, "VISA":refnum<visa-resource-name>, "enable 10MHz ref":bool, "cmi ckd2":T21, "cmi sync v3":T24, "trigger":T33, "HMF2500 cfg":T37}
  T20 = typedef "AWG.lvlib/AWG Type.ctl" = enum16{"Agilent 331xxA to 332xxA", "Agilent 335xxA to 336xxA", "Tektronix AFG3101C", "R&S HMF25xx", "CMI Clock Divider v2", "CMI Sync Unit V3", "dummy"}
  T21 = typedef "AWG.lvlib/CMI ckd2 Session.ctl" = cluster{"VISA":refnum<visa-resource-name>, "clock source":T22, "manual ref clk":bool, "ref clock [Hz]":dbl, "div mode":T23}
  T22 = typedef "AWG.lvlib/CMI ckd2 Source Mode.ctl" = enum16{"Auto", "LF clock", "HF clock", "Internal"}
  T23 = typedef "AWG.lvlib/CMI ckd2 Divisor Mode.ctl" = enum16{"Set divisor directly", "Set divisor by frequency"}
  T24 = typedef "AWG.lvlib/CMI Sync Unit V3.lvlib/CMI Sync V3 session.ctl" = cluster{"VISA":refnum<visa-resource-name>, "baud rate [bd/s]":i32, "source":T25, "hv range":T26, "fsrc is fixed":bool, "fsrc [Hz]":dbl, "freq integ [s]":dbl, "freq filter":i32, "trig level":T27, "chn1 mode":T28, "chn1 level":T29, "chn2 mode":T30, "chn2 level":T29, "chn2 div":i32, "chn3 mode":T31, "chn3 level":T29, "chn1 div entry":T32, "chn1 dev limit [%]":dbl, "chn1 check dev":bool}
  T25 = typedef "AWG.lvlib/CMI Sync Unit V3.lvlib/CMI Sync V3 Reference Clock Source.ctl" = enum16{"Auto", "Internal", "Logic", "Sine", "HV"}
  T26 = typedef "AWG.lvlib/CMI Sync Unit V3.lvlib/CMI Sync V3 HV input Range.ctl" = enum16{"10V", "60V", "250V", "1kV"}
  T27 = typedef "AWG.lvlib/CMI Sync Unit V3.lvlib/CMI Sync V3 Trigger Input Level.ctl" = enum16{"LVCMOS 3V3", "TTL 5V"}
  T28 = typedef "AWG.lvlib/CMI Sync Unit V3.lvlib/CMI Sync V3 Channel 1 Mode.ctl" = enum16{"Source divider", "DDS absolute", "DDS ratio", "DDS ratio M/N"}
  T29 = typedef "AWG.lvlib/CMI Sync Unit V3.lvlib/CMI Sync V3 Channel Output Levels.ctl" = enum16{"Positive 3V3", "Negative 3V3", "Positive 5V", "Negative 5V"}
  T30 = typedef "AWG.lvlib/CMI Sync Unit V3.lvlib/CMI Sync V3 Channel 2 Mode.ctl" = enum16{"Source divider", "Chn 1 divide"}
  T31 = typedef "AWG.lvlib/CMI Sync Unit V3.lvlib/CMI Sync V3 Channel 3 Mode.ctl" = enum16{"Chn 1 Active", "Chn 2 Active", "Chn 1 Trigger", "Chn 2 Trigger", "Gate", "PPS", "10MHz"}
  T32 = typedef "AWG.lvlib/CMI Sync Unit V3.lvlib/CMI Sync V3 Channel 1 Divisor Entry Mode.ctl" = enum16{"Set divisor directly", "Calculate nearest divisor from measured fx"}
  T33 = typedef "ADC Trig Config.ctl" = cluster{"source":T34, "slope":T35, "coupling":T36, "level [V]":dbl, "hysteresis [V]":dbl, "pre-trigger [%]":dbl}
  T34 = typedef "ADC Trig Mode Source.ctl" = enum16{"Immediate", "External", "Level"}
  T35 = typedef "ADC Trig Slope.ctl" = enum16{"POS", "NEG"}
  T36 = typedef "ADC Trig Coupling.ctl" = enum16{"DC", "AC"}
  T37 = typedef "AWG.lvlib/HMF2500 Config.ctl" = cluster{"Baud Rate":u32, "Parity":u16, "Data Bits":u16, "Flow Control":u16}
  T38 = typedef "3458A Virtual Digitizer.lvlib/3458A Sync Mode.ctl" = enum16{"MASTER-SLAVE, MASTER clocked by TIMER", "MASTER-SLAVE, MASTER clocked by AWG", "ALL clocked by AWG", "MASTER-SLAVE, ALL clocked by TIMER", "ALL clocked by AWG with DFLL"}
  T39 = typedef "3458A Virtual Digitizer.lvlib/3458A Idn Mode.ctl" = enum16{"Auto", "Sequential (chn A, chn B, ...)", "From calibration string"}
  T40 = typedef "3458A Virtual Digitizer.lvlib/3458A Digitizing Low Levels.lvlib/Sampling Mode.ctl" = enum16{"DCV", "DSDC", "DSAC"}
  T41 = typedef "3458A Virtual Digitizer.lvlib/3458A Digitizing Process Options.ctl" = cluster{"channel id":i32, "packet size [smpl]":i32, "current timeout [s]":dbl, "blk2blk timeout [s]":dbl, "event time":timestamp, "stop notifier":refnum<notifier>, "data queues":refnum<queue>[], "proc refs":refnum<vi>[], "bus semaphore":T42}
  T42 = typedef "Semaphore RefNum" = refnum<k1>
  T43 = typedef "3458A Virtual Digitizer.lvlib/3458A Aux Record Data.ctl" = cluster{"channel id":i32, "valid?":bool[], "gain [V]":dbl[], "timestamp [s]":dbl[], "Ts [s]":dbl, "abs timestamp":timestamp, "t [deg C]":dbl[], "multiplex timestamp [s]":dbl, "only multiplex?":bool, "multiplex smpl offset":i64, "overflow?":bool}
  T44 = typedef "3458A Virtual Digitizer.lvlib/3458A Digitizing Low Levels.lvlib/Level Setup.ctl" = cluster{"edge":enum16{"POS", "NEG"}, "level [V]":dbl, "coupling":enum16{"DC", "AC"}}
  T45 = typedef "3458A Virtual Digitizer.lvlib/3458A Digitizing Low Levels.lvlib/First Sample Trigger.ctl" = enum16{"AUTO", "EXT", "SYN", "SGL", "HOLD", "LEVEL"}
  T46 = typedef "3458A Virtual Digitizer.lvlib/3458A Aperture Selection Mode.ctl" = enum16{"Manual", "Maximum", "Table"}
  T47 = typedef "3458A Virtual Digitizer.lvlib/3458A Multiplexing Config.ctl" = cluster{"cycles":i32, "delay [s]":dbl, "enabled":bool, "overhead [s]":dbl, "tot smpls":i64, "sub-rec":i32, "overhead [%]":dbl, "emulated":bool}
  T48 = typedef "F8588A Low Pass Filter.ctl" = enum16{"Off", "100 kHz", "3 MHz"}
  T49 = typedef "F8588A Phase Lock.ctl" = enum16{"Off", "1 MHz", "10 MHz"}
  T50 = typedef "F8588A Coupling.ctl" = enum16{"AC, 1 MOhm", "AC, 10 MOhm", "DC, 1 MOhm", "DC, 10 MOhm", "DC, auto"}
  T51 = typedef "3458A Virtual Digitizer.lvlib/3458A Sampling Rate.ctl" = cluster{"freq mode":T52, "fs [Hz]":dbl, "fref [Hz]":dbl, "mul":dbl, "div":dbl}
  T52 = typedef "AWG.lvlib/AWG Clock Setup Mode.ctl" = enum16{"fs or Ts", "fs or Ts with fref", "fref/N", "fref*M/N", "fref*Ratio"}
  T53 = typedef "3458A Sample Rate Mode.ctl" = enum16{"fs or Ts", "fs*M/N"}
  T54 = typedef "DSDLL Virtual Digitizer.lvlib/DSDLL Session.ctl" = cluster{"dsdll":T55, "channels":i32, "device id":i32, "channel idns":string[], "proc setup":T57, "samples count":i32, "fs [Hz]":dbl}
  T55 = typedef "dsdll.lvlib/dsdll_instance.ctl" = cluster{"dsdll path":path, "dsdll handle":u8[], "output devices":T56[], "capture devices":T56[]}
  T56 = typedef "dsdll.lvlib/dsdll_device_record.ctl" = cluster{"guid":u8[], "name":string}
  T57 = typedef "DSDLL Virtual Digitizer.lvlib/DSDLL Process Config.ctl" = cluster{"packet size [smpl]":i32, "current timeout [s]":dbl, "blk2blk timeout [s]":dbl, "event time":timestamp, "data queue":refnum<queue>, "stop notifier":refnum<notifier>, "proc ref":refnum<vi>}
  T58 = typedef "ADC Type.ctl" = enum16{"niScope", "3458A", "DirectSound DLL", "Keysight DSO", "cDAQ ADC", "CMI ADS127L21", "dummy"}
  T59 = typedef "SimAdc Config.ctl" = cluster{"channels":T60[], "range [V]":dbl, "Ts step [s]":dbl, "time [s]":dbl, "fs [Hz]":dbl, "count":i64, "smpl offset":i64, "set count":i64, "bit res":i32}
  T60 = typedef "SimAdc Channel Cfg.ctl" = cluster{"harmonics":dbl[][], "btn clear":bool, "noise":dbl, "fundamental [Hz]":dbl}
  T61 = typedef "ADC On Close Action.ctl" = enum16{"Immediate reset", "Delayed reset"}
  T62 = typedef "MPX Session.ctl" = cluster{"Type":T63, "gen com ssn":T64, "delay before [s]":dbl, "delay post [s]":dbl, "sequence":string[], "enabled":bool, "ref timestamp [s]":dbl, "idn string":string, "dev niScope":refnum<k15>, "niScope idx":i32, "QPMX ssn":T68, "VISA mux ssn":T71}
  T63 = typedef "MPX Type.ctl" = enum16{"Dummy", "Generic - COM port", "Generic - niScope PFI", "Generic - VISA commands", "QPMX"}
  T64 = typedef "GCOMM Session.ctl" = cluster{"visa":refnum<visa-resource-name>, "primary":T65, "secondary":T65, "channels":T66[]}
  T65 = typedef "GCOMM Signal.ctl" = enum16{"None", "DTR", "RTS"}
  T66 = typedef "GCOMM Virtual Channel.ctl" = cluster{"Primary:":T67, "Secondary:":T67, "btn clr":bool, "btn up":bool, "btn down":bool, "Tag:":string}
  T67 = typedef "GCOMM Logic State.ctl" = enum16{"OFF", "ON"}
  T68 = typedef "QPMX Session.ctl" = cluster{"visa":refnum<visa-resource-name>, "switch mode":T69, "sequence":bool[][], "timing delays":u32[], "polarity":T70, "ss delay (s)":dbl, "internal timer (s)":dbl, "Last loaded sequence file":path, "startup delay (s)":dbl}
  T69 = typedef "QPMX switch mode.ctl" = enum16{"Switched by TWM", "Switched by external clock", "Switched by internal clock"}
  T70 = typedef "QPMX polarity.ctl" = enum16{"Positive", "Negative"}
  T71 = typedef "GVISA Mux Session.ctl" = cluster{"VISA":refnum<visa-resource-name>, "paths":T72[], "idn command":string, "serial cfg":T73}
  T72 = typedef "GVISA Mux Path Entry.ctl" = cluster{"Tag:":string, "Command:":string, "btn clr":bool, "btn up":bool, "btn down":bool}
  T73 = typedef "met_serial_setup.ctl" = cluster{"Baud rate":i32, "Data bits":i32, "Parity":i32, "Stop bits":i32, "Flow control":i32, "End Mode Read":enum16{"None", "Last Bit", "TermChar"}, "End Mode Write":enum16{"None", "Last Bit", "TermChar"}, "Term character":u8, "Term enable":bool}
  T74 = typedef "KeDSO session.ctl" = cluster{"VISA":refnum<visa-resource-name>, "channels":T75[], "bw limit [Hz]":dbl, "resolution":T76, "trig noise reject":enum16{"Normal", "High Sensitivity"}, "N":i64, "trigger config":T77, "fs [Hz]":dbl, "timeout stop":timestamp, "waiting for opc":bool, "fetch offset [smpl]":i64, "abs timestamp":timestamp, "ranges [V]":dbl[], "decimation":dbl, "ext ref":bool, "emulate aperture":bool, "model":T79}
  T75 = typedef "KeDSO Virtual Channel.ctl" = cluster{"Channel":i32, "Range [Vpk]":dbl, "btn clr":bool, "btn up":bool, "btn down":bool, "Offset [V]":dbl, "Coupling":enum16{"DC", "DC50", "AC", "LFR1"}, "bw limit enab":bool}
  T76 = typedef "KeDSO High Resolution Mode.ctl" = enum16{"Basic", "High-res AUTO", "Min. 9-bits", "Min. 10-bits", "Min. 11-bits", "Min. 12-bits", "Fixed 11-bits", "Fixed 12-bits", "Fixed 13-bits", "Fixed 14-bits", "Fixed 15-bits", "Fixed 16-bits"}
  T77 = typedef "KeDSO Trigger Setup.ctl" = cluster{"trigger source":T78, "trigger slope":enum16{"Negative", "Positive", "Either"}, "level [V]":dbl, "hysteresis [V]":dbl, "pre-trig [%]":i32}
  T78 = typedef "KeDSO Trigger Source.ctl" = enum16{"Immediate", "Level", "AUX"}
  T79 = typedef "Agilent 90000 Series.lvlib/DSO type.ctl" = enum16{"DSO91304", "DSO91204", "DSO90804", "DSO90604", "DSO90404", "DSO90254", "DSA91304", "DSA91204", "DSA90804", "DSA90604", "DSA90404", "DSA90254", "DSO9104", "DSO9254", "DSO9404", "MSO9104", "MSO9254", "MSO9404", "MSO9064", "DSO9064", "DSOX91604", "DSOX92004", "DSOX92504", "DSOX92804", "DSOX93204", "DSO93004", "DSO9024H", "DSO9054H", "DSO9104H", "DSO9204H", "DSOS054A", "DSOS104A", "DSOS204A", "DSOS254A", "DSOS404A", "DSOS604A", "DSOS804A", "MSOS054A", "MSOS104A", "MSOS204A", "MSOS254A", "MSOS404A", "MSOS604A", "MSOS804A", "DSAX96204Q", "DSOX96204Q", "DSAX95004Q", "DSOX95004Q", "DSAX93304Q", "DSOX93304Q", "DSAX92504Q", "DSOX92504Q", "DSAX92004Q", "DSOX92004Q"}
  T80 = typedef "cDAQ Session.ctl" = cluster{"mclk [Hz]":dbl, "ADC task":refnum<k21>, "mclk reference":string, "fs [Hz]":dbl, "queue adc cmd":refnum<queue>, "queue adc data":refnum<queue>, "adc proc ref":refnum<vi>, "channels":T81[], "last channels":T81[], "timeout":timestamp, "N":i32, "mclk mode":T82, "ext mclk source":tag}
  T81 = typedef "cDAQ Virtual Channel.ctl" = cluster{"Device":tag, "Channel id":i32, "btn clr":bool, "btn up":bool, "btn down":bool}
  T82 = typedef "cDAQ Master Clock Mode.ctl" = enum16{"Free running", "Export master clock", "Import master clock"}
  T83 = typedef "CMI ADS127L21 - Session.ctl" = cluster{"VISA":refnum<visa-resource-name>, "chn list":i32[], "record size":i32, "phys. channels":i32, "adc fifo size":i32, "channels":T84[], "ext refclk?":bool, "fs [Hz]":dbl, "ext refclk [Hz]":dbl, "meas refclk [Hz]":dbl, "EXTOUT mode":T88, "EXTOUT polarity":T89, "EXTOUT divisor":i32}
  T84 = typedef "CMI ADS127L21 - Record Channel.ctl" = cluster{"Range [Vpk]":T85, "Channel":i32, "Mode":T86, "Impedance":T87, "btn clr":bool, "btn up":bool, "btn down":bool}
  T85 = typedef "CMI ADS127L21 - Input Range.ctl" = dbl
  T86 = typedef "CMI ADS127L21 - Input Mode.ctl" = enum16{"Normal", "Inverted", "GND"}
  T87 = typedef "CMI ADS127L21 - Input Impedance.ctl" = enum16{"1M", "1k5"}
  T88 = typedef "CMI ADS127L21 - EXTOUT Mode.ctl" = enum16{"ADCCLK", "REFCLK", "SMPLCLK", "FIRST"}
  T89 = typedef "CMI ADS127L21 - EXTOUT Polarity.ctl" = enum16{"NORM", "INV"}
  T90 = typedef "Meas Sequence Item.ctl" = cluster{"config":T91, "data file path":path, "header file path":path, "group id":i32, "rec id":i32, "group done?":bool, "adc modified?":bool, "source modified?":bool, "progress [%]":dbl, "groups cnt":i32, "rec cnt":i32, "data file relative path":string, "meas root path":path, "calculate?":bool, "comment":string, "avg cnt":i32}
  T91 = typedef "Meas Sampling Configuration.ctl" = cluster{"count [smpl]":i64, "aperture [s]":dbl, "trigger":T33, "ranges [Vpk]":dbl[], "QWTB parameters":T92[], "sampling rate":T51}
  T92 = typedef "Meas Proc QWTB Algorithm Parameter Data.ctl" = cluster{"name":string, "numerics":dbl[], "strings":string[]}
  T93 = typedef "Meas Sequence Configuration.ctl" = cluster{"group setups":T91[], "rec count":i32, "range mode":T94, "fs mode":T95, "rng even":dbl, "rng odd":dbl, "folder":path, "name base":string, "meas id":i32, "settle [s]":dbl, "comment":string, "avg count":i32, "fs-abs-fr fr":dbl, "fs-abs-fr fs":dbl, "fs-div fr":dbl, "fs-div div":dbl, "fs-mn fr":dbl, "fs-mn mul":dbl, "fs-mn div":dbl, "fs-rat fr":dbl, "fs-rat rat":dbl}
  T94 = typedef "Meas Range Mode.ctl" = enum16{"Keep defaults", "Set All channels", "Set Odd and Even channels"}
  T95 = typedef "Meas Sampling Rate Mode.ctl" = enum16{"Frequency", "Period"}
  T96 = typedef "Meas Process Config.ctl" = cluster{"mode":T97, "call after avgs?":bool, "calculate?":bool, "raw mode":T98, "QWTB":T100}
  T97 = typedef "Meas Process Mode.ctl" = enum16{"Raw", "QWTB"}
  T98 = typedef "Meas Process Raw Config.ctl" = cluster{"command":string, "result mode":T99, "res variable":string}
  T99 = typedef "Meas Process Raw Result Mode.ctl" = enum16{"Display console output (only Octave)", "Display string variable", "Display result file %respath%"}
  T100 = typedef "Meas Proc QWTB Setup.ctl" = cluster{"QWTB path":path, "alg filter path":string, "alg ids":string[], "alg parameters":string[], "parsed parameters":T92[], "selected alg id":string, "selected unc mode":T101, "qwtb mcc":i32, "qwtb timeout":i32, "qwtb covg":dbl, "qwtb ofs":i64, "qwtb lim data":i64, "multicore":T102, "unc once?":bool, "qwtb tstemp":T104, "octave reset":bool, "exec mode":T105}
  T101 = typedef "Meas Proc QWTB Uncertainty Mode.ctl" = enum16{"None", "GUF", "Monte Carlo"}
  T102 = typedef "Meas Proc QWTB Multicore Setup.ctl" = cluster{"jobs folder":path, "cores":i32, "max jobs":i32, "mode":T103}
  T103 = typedef "Meas Proc QWTB Multicore Type.ctl" = enum16{"Singlecore", "Multicore", "Multistation"}
  T104 = typedef "Meas Process Time Stamp Mode.ctl" = enum16{"Enabled (default)", "Disabled", "Relative to 1. record"}
  T105 = typedef "Meas Proc QWTB Exec Mode.ctl" = enum16{"Single-core", "Parallel Record Processing"}
  T106 = typedef "Corr Setup.ctl" = cluster{"transducers":cluster{"channels":T107[], "last path":path, "root path":path}, "digitizer":T108}
  T107 = typedef "Corr Tranducer Item.ctl" = cluster{"Path":path, "Ratio:":string, "Name:":string, "btn rem":bool, "btn up":bool, "btn down":bool, "s.n.:":string, "btn open":bool, "ratio o/i":dbl, "chn hi":u16, "chn lo":u16, "Phase index":i32, "btn edit":bool, "mpx chn":u16, "btn vdx1":bool, "btn csx1":bool, "invert":bool}
  T108 = typedef "Corr Digitizers.ctl" = cluster{"last path":path, "channel paths":path[], "channel idns":string[], "correction name":string, "channel names":string[], "folders to copy":path[], "channel valid":bool[], "correction path":path, "correction rel path":string, "rel folders to copy":string[], "root path":path}
  T109 = typedef "Assist Panel Setup.ctl" = cluster{"P":i32, "Q":i32, "rel shift":dbl, "ref freq":dbl, "min fs":dbl, "max fs tol":dbl, "min int":dbl, "max int":dbl, "max err":dbl, "max timeout":dbl}
  T110 = typedef "varilib.lvlib/SGUI Assign References Mode.ctl" = enum16{"Add to stack", "Overwrite", "Release last", "Release ID"}
  T111 = typedef "GOLPI library.lvlib/GOLPI reference Type Def.ctl" = cluster{"pipe handle":T112, "fast read timeout [ms]":u32, "fast read settle time [ms]":u32, "fast read to multiple [ms]":u32, "max elements per input line":u32, "slow read timeout [ms]":u32, "stdin double format specifier":string, "max elements per stdout output column":u32, "console mode bitstream":bool, "bitstream first read timeout [ms]":u32, "bitstream read timeout [ms]":u32, "struct transfer possible":bool, "matlab mode":bool}
  T112 = typedef "LV Process library.lvlib/Pipe Handle.ctl" = cluster{"lv_proc.dll file path":path, "process instance handle":u32[], "debug mode":bool, "debug data":cluster{"time":timestamp, "stdin":bool, "data":string}[]}
  T113 = typedef "GOLPI Multi Process.lvlib/golpi_session.ctl" = cluster{"GOLPI ref":T111, "idn str":string, "octave path":path, "work path":path, "start timeout [ms]":u32, "clr cache":bool, "console":bool, "binary":bool, "semaphore":T42, "initial command":string, "exit command":string, "matlab":bool, "pkg list":string[]}
  T114 = typedef "LVPointTypeDef.ctl" = cluster{"Horizontal":i16, "Vertical":i16}
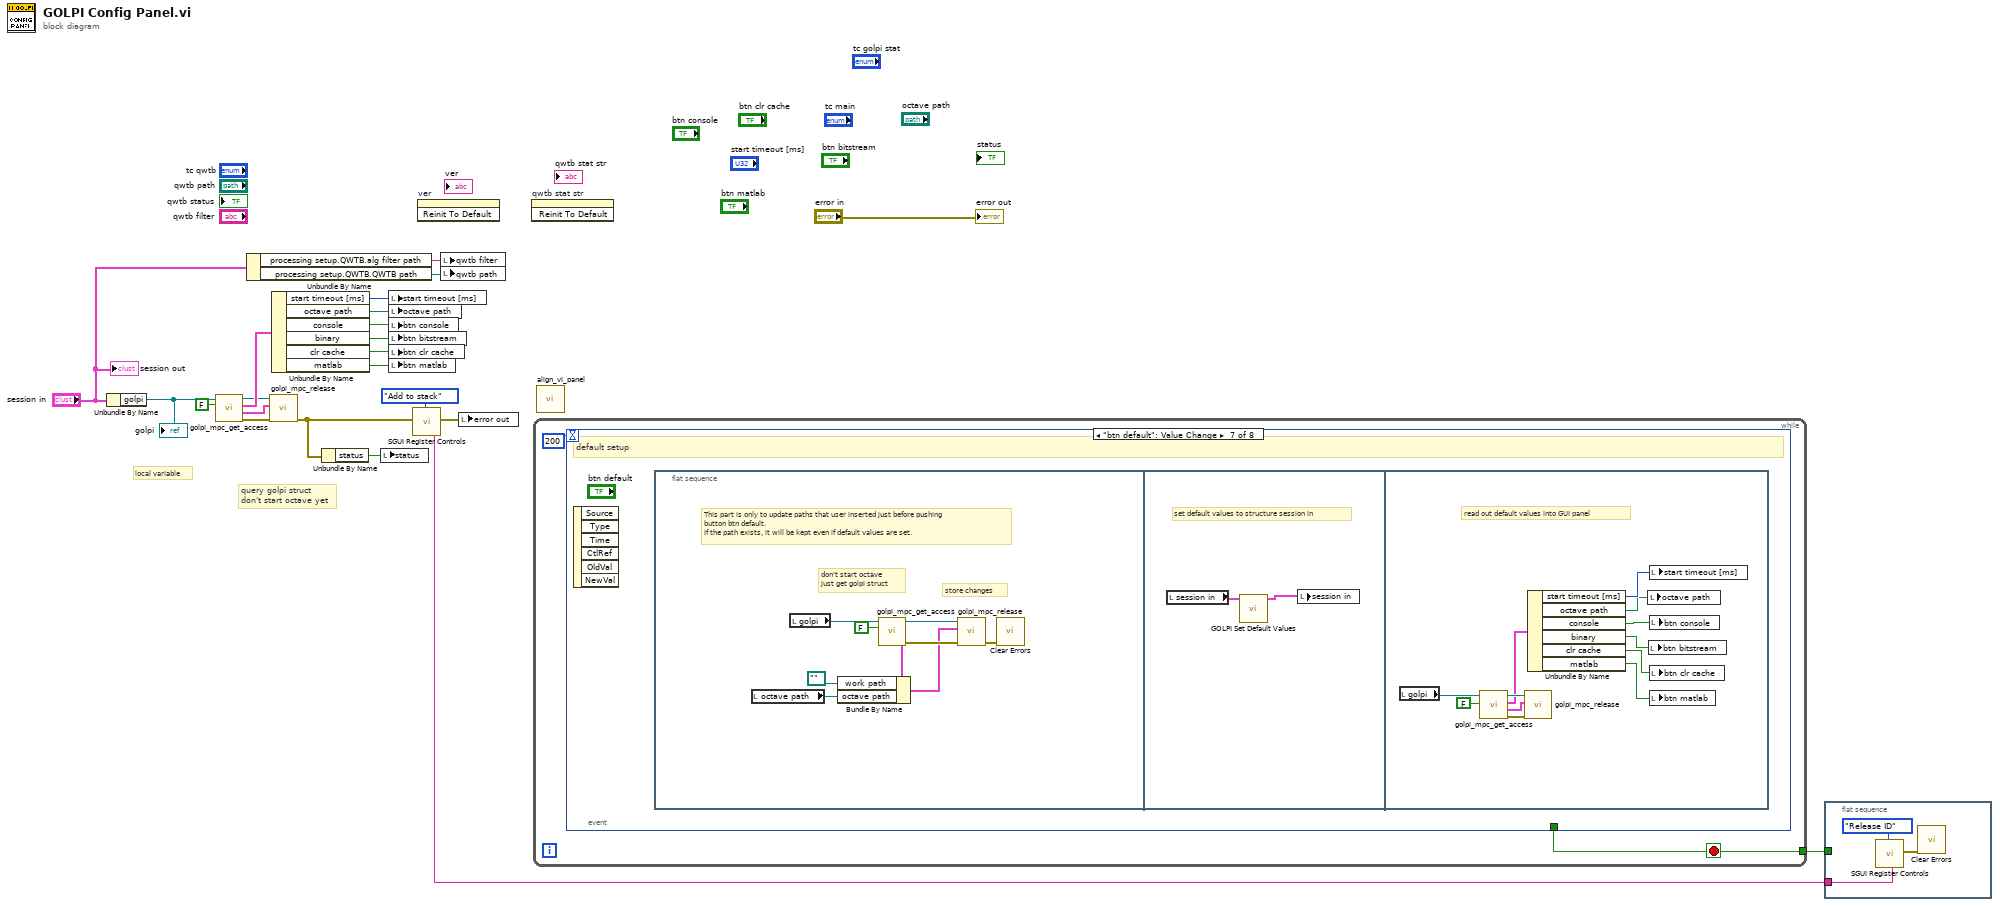
[diagram p0: block diagram]
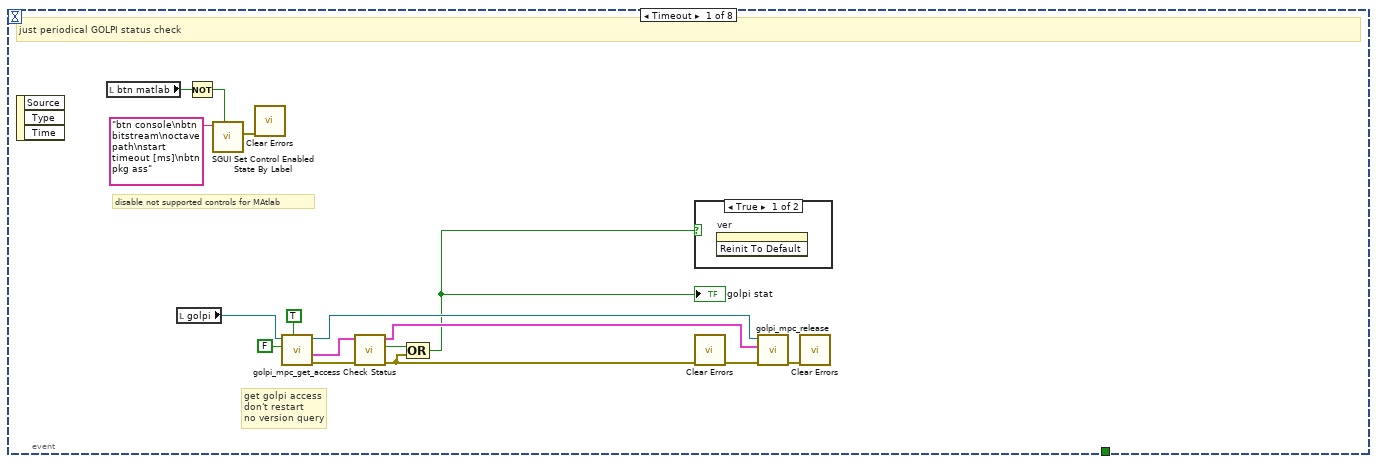
[diagram p2: hidden frame]
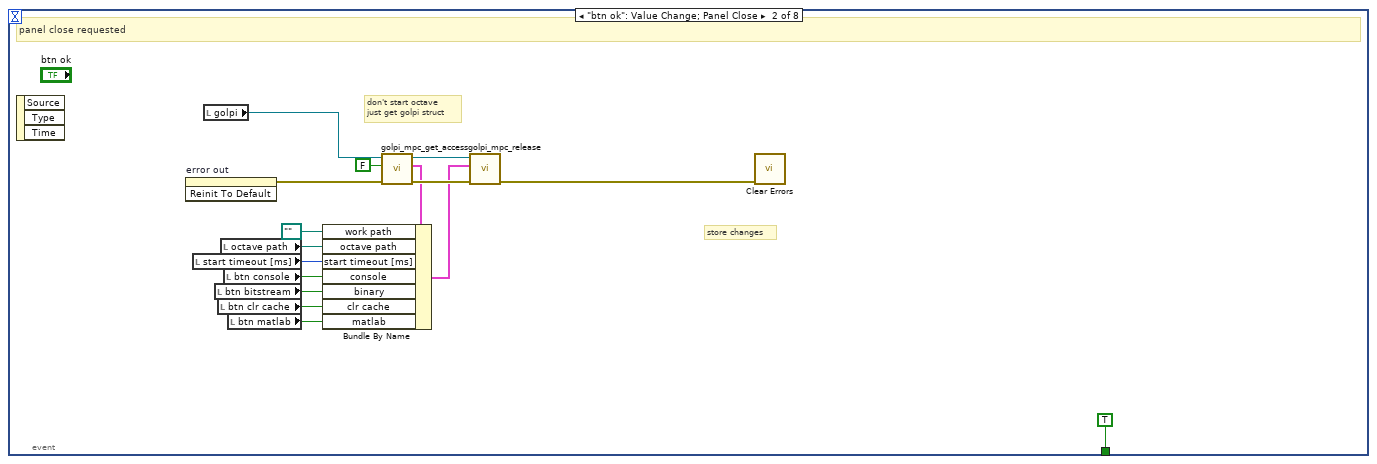
[diagram p4: hidden frame]
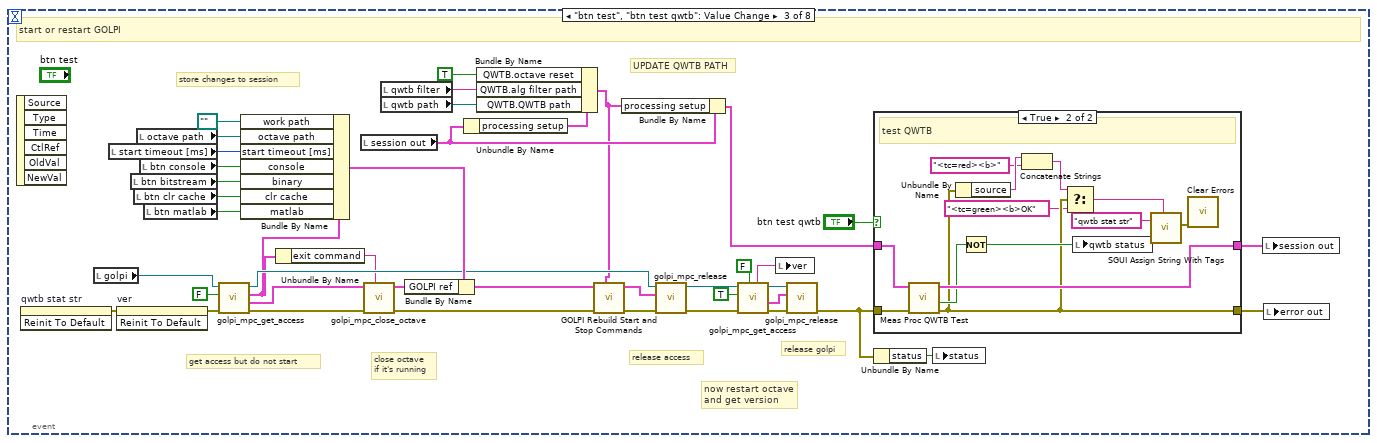
[diagram p5: hidden frame]
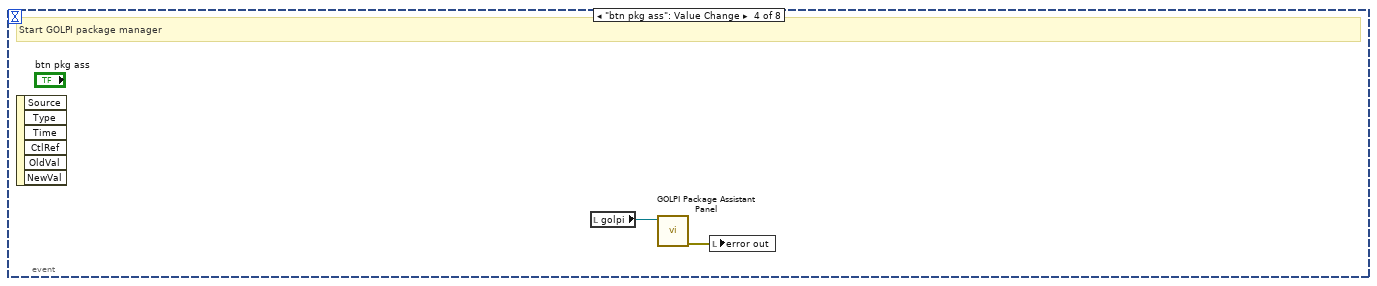
[diagram p7: hidden frame]
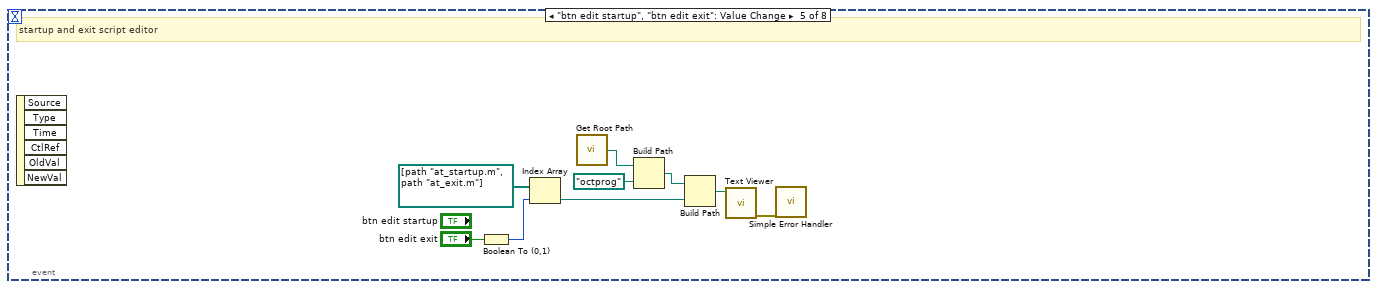
[diagram p8: hidden frame]
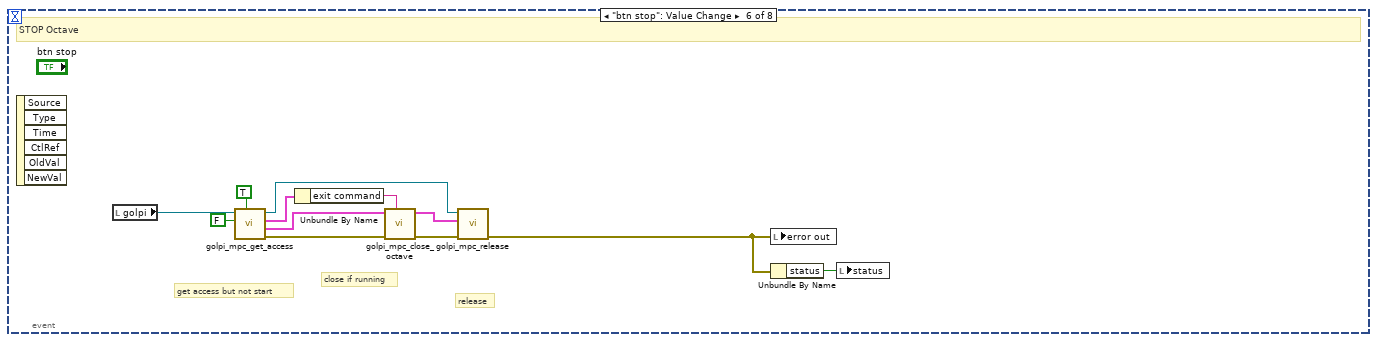
[diagram p9: hidden frame]
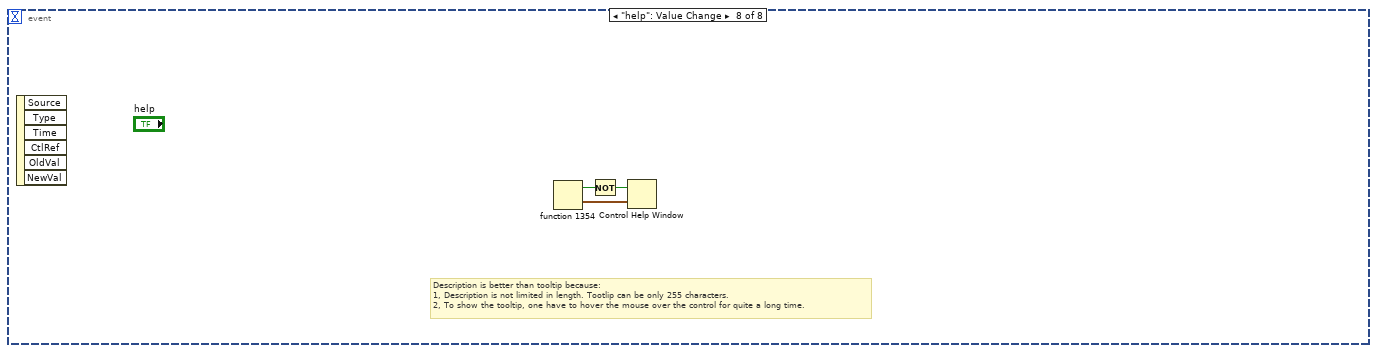
[diagram p10: hidden frame]
diagram:
  # "local variable"
  # "query golpi struct\ndon't start octave yet"
  n1 = Unbundle By Name("session in") -> ("golpi"=w10:T1)
  "golpi" <- w10
  n2 = call "golpi_mpc_get_access.vi"("allow octave start (true)"=FALSE, "golpi session ref"=w10) -> ("error out"=w17:errorcluster, "GOLPI ref out"=w14:T111, "golpi session out"=w16:T113, "golpi session ref out (copy)"=w15:T1)  [unwired: 4 in, 2 out]
  n3 = Unbundle By Name("session in") -> ("processing setup.QWTB.alg filter path"=w7:string, "processing setup.QWTB.QWTB path"=w8:path)
  n4 = call "golpi_mpc_release.vi"("error in"=w17, "golpi ref or golpi session in"=w14, "golpi session ref"=w15) -> ("error out"=w6:errorcluster)  [unwired: 7 in, 1 out]
  n5 = Unbundle By Name(w16) -> ("start timeout [ms]"=w21:u32, "octave path"=w20:path, "console"=w19:bool, "binary"=w12:bool, "clr cache"=w11:bool, "matlab"=w2:bool)
  n6 = Unbundle By Name(w6) -> ("status"=w18:bool)
  n7 = local write "status"(w18) -> ()
  n8 = local write "start timeout [ms]"(w21) -> ()
  n9 = local write "octave path"(w20) -> ()
  n10 = local write "btn console"(w19) -> ()
  n11 = local write "btn bitstream"(w12) -> ()
  n12 = local write "btn clr cache"(w11) -> ()
  n13 = local write "btn matlab"(w2) -> ()
  n14 = call "SGUI Register Controls.vi"("error in"=w6, "register mode (overwrite)"=SGUI_Assign_References_Mode."Add to stack") -> ("assigned ID"=w1:string, "error out"=w5:errorcluster)  [unwired: 15 in, 1 out]
  n15 = invoke on="ver" class="Str" method="Reinit To Default"() -> ()  [unwired: 3 in, 3 out]
  n16 = local write "qwtb filter"(w7) -> ()
  n17 = local write "qwtb path"(w8) -> ()
  n18 = local write "error out"(w5) -> ()
  n19 = invoke on="qwtb stat str" class="Str" method="Reinit To Default"() -> ()  [unwired: 3 in, 3 out]
  n20 = while {
    tunnel: [w23] -> w3
    stop <- w23 stop-if-true
    n21 = event shown="[6] \"btn default\": Value Change" {
      selector: _ -> [_ _ _ _ _ _ _ _]
      dyn-events: _ -> [_ _ _ _ _ _ _ _]
      timeout: 200 -> [_ _ _ _ _ _ _ _]
      tunnel: [_ TRUE _ _ _ _ _ _] -> w23
      event Timeout {
        # "disable not supported controls for MAtlab"
        # "get golpi access\ndon't restart\nno version query"
        # "just periodical GOLPI status check"
        n22 = event-data() -> ()  [unwired: 1 in, 3 out]
        n23 = local read "btn matlab"() -> (w28:bool)
        n24 = local read "golpi"() -> (w37:T1)
        n25 = Not(x=w28) -> (.not. x?=w26:bool)
        n26 = call "SGUI Set Control Enabled State By Label.vi"("labels (empty)"="btn console\nbtn bitstream\noctave path\nstart timeout [ms]\nbtn pkg ass", "Enabled? (False)"=w26) -> ("error out"=w25:errorcluster)  [unwired: 8 in, 1 out]
        n27 = call <vilib>:"Clear Errors.vi"("error in (no error)"=w25) -> ()  [unwired: 5 in, 2 out]
        n28 = call "golpi_mpc_get_access.vi"("don't query version (true)"=TRUE, "allow octave start (true)"=FALSE, "golpi session ref"=w37) -> ("error out"=w40:errorcluster, "GOLPI ref out"=w39:T111, "golpi session ref out (copy)"=w35:T1)  [unwired: 3 in, 3 out]
        n29 = call "Check Status.vi"("error in"=w40, "GOLPI ref. in"=w39) -> ("error out"=w32:errorcluster, "exited?"=w31:bool, "GOLPI ref. out"=w34:T111)  [unwired: 7 in]
        n30 = Compound Arithmetic op=OR(w31, w32) -> (w30:bool)
        "golpi stat" <- w30
        n31 = case shown="True" w30 {
          frame True {
            n32 = invoke on="ver" class="Str" method="Reinit To Default"() -> ()  [unwired: 3 in, 3 out]
          }
          frame False {
          }
        }
        n33 = call <vilib>:"Clear Errors.vi"("error in (no error)"=w32) -> ("error out"=w36:errorcluster)  [unwired: 5 in, 1 out]
        n34 = call "golpi_mpc_release.vi"("error in"=w36, "golpi ref or golpi session in"=w34, "golpi session ref"=w35) -> ("error out"=w29:errorcluster)  [unwired: 7 in, 1 out]
        n35 = call <vilib>:"Clear Errors.vi"("error in (no error)"=w29) -> ()  [unwired: 5 in, 2 out]
      }
      event "btn ok": Value Change; Panel Close {
        # "store changes"
        # "don't start octave\njust get golpi struct"
        # "panel close requested"
        n36 = event-data() -> ()  [unwired: 1 in, 3 out]
        n37 = invoke on="error out" class="Clust (strict)" method="Reinit To Default"() -> (error out=w43:errorcluster)  [unwired: 3 in, 2 out]
        n38 = local read "start timeout [ms]"() -> (w55:u32)
        n39 = local read "golpi"() -> (w50:T1)
        n40 = local read "btn bitstream"() -> (w45:bool)
        n41 = local read "btn clr cache"() -> (w44:bool)
        n42 = local read "octave path"() -> (w53:path)
        n43 = local read "btn console"() -> (w54:bool)
        n44 = local read "btn matlab"() -> (w42:bool)
        n45 = call "golpi_mpc_get_access.vi"("error in"=w43, "allow octave start (true)"=FALSE, "golpi session ref"=w50) -> ("error out"=w52:errorcluster, "golpi session out"=w49:T113, "golpi session ref out (copy)"=w51:T1)  [unwired: 3 in, 3 out]
        n46 = Bundle By Name(cluster=w49, "work path"=path "", "octave path"=w53, "start timeout [ms]"=w55, "console"=w54, "binary"=w45, "clr cache"=w44, "matlab"=w42) -> (w48:T113)
        n47 = call "golpi_mpc_release.vi"("error in"=w52, "golpi ref or golpi session in"=w48, "golpi session ref"=w51) -> ("error out"=w47:errorcluster)  [unwired: 7 in, 1 out]
        n48 = call <vilib>:"Clear Errors.vi"("error in (no error)"=w47) -> ()  [unwired: 5 in, 2 out]
      }
      event "btn test", "btn test qwtb": Value Change {
        # "UPDATE QWTB PATH"
        # "get access but do not start"
        # "store changes to session"
        # "release golpi"
        # "now restart octave\nand get version"
        # "release access"
        # "close octave\nif it's running"
        # "start or restart GOLPI"
        n49 = event-data() -> ()  [unwired: 1 in, 6 out]
        n50 = invoke on="qwtb stat str" class="Str" method="Reinit To Default"() -> (error out=w63:errorcluster)  [unwired: 3 in, 2 out]
        n51 = local read "golpi"() -> (w83:T1)
        n52 = local read "start timeout [ms]"() -> (w97:u32)
        n53 = invoke on="ver" class="Str" method="Reinit To Default"(error in=w63) -> (error out=w85:errorcluster)  [unwired: 2 in, 2 out]
        n54 = local read "btn bitstream"() -> (w87:bool)
        n55 = local read "btn clr cache"() -> (w86:bool)
        n56 = local read "octave path"() -> (w95:path)
        n57 = local read "btn console"() -> (w96:bool)
        n58 = local read "btn matlab"() -> (w59:bool)
        n59 = call "golpi_mpc_get_access.vi"("error in"=w85, "allow octave start (true)"=FALSE, "golpi session ref"=w83) -> ("error out"=w84:errorcluster, "GOLPI ref out"=w81:T111, "golpi session out"=w76:T113, "golpi session ref out (copy)"=w77:T1)  [unwired: 3 in, 2 out]
        n60 = Bundle By Name(cluster=w76, "work path"=path "", "octave path"=w95, "start timeout [ms]"=w97, "console"=w96, "binary"=w87, "clr cache"=w86, "matlab"=w59) -> (w80:T113)
        n61 = Unbundle By Name(w76) -> ("exit command"=w75:string)
        n62 = local read "session out"() -> (w69:T2)
        n63 = call "golpi_mpc_close_octave.vi"("exit command (empty)"=w75, "error in"=w84, "GOLPI ref in"=w81) -> ("error out"=w74:errorcluster, "GOLPI ref out (empty)"=w79:T111)  [unwired: 6 in, 1 out]
        n64 = local read "qwtb filter"() -> (w60:string)
        n65 = local read "qwtb path"() -> (w61:path)
        n66 = Bundle By Name(cluster=w80, "GOLPI ref"=w79) -> (w73:T113)
        n67 = Unbundle By Name(w69) -> ("processing setup"=w70:T96)
        n68 = Bundle By Name(cluster=w70, "QWTB.octave reset"=TRUE, "QWTB.alg filter path"=w60, "QWTB.QWTB path"=w61) -> (w68:T96)
        n69 = call "GOLPI Rebuild Start and Stop Commands.vi"("processing setup"=w68, "error in"=w74, "golpi session in"=w73) -> ("error out"=w72:errorcluster, "golpi session out"=w71:T113)  [unwired: 7 in]
        n70 = Bundle By Name(cluster=w69, "processing setup"=w68) -> (w66:T2)
        n71 = call "golpi_mpc_release.vi"("error in"=w72, "golpi ref or golpi session in"=w71, "golpi session ref"=w77) -> ("error out"=w94:errorcluster, "golpi session out (copy)"=w93:T1)  [unwired: 7 in]
        n72 = call "golpi_mpc_get_access.vi"("don't query version (true)"=FALSE, "error in"=w94, "allow octave start (true)"=TRUE, "golpi session ref"=w93) -> ("error out"=w91:errorcluster, "GOLPI ref out"=w89:T111, "golpi session ref out (copy)"=w90:T1, "GNU Octave version"=w88:string)  [unwired: 2 in, 2 out]
        n73 = local write "ver"(w88) -> ()
        n74 = call "golpi_mpc_release.vi"("error in"=w91, "golpi ref or golpi session in"=w89, "golpi session ref"=w90) -> ("error out"=w62:errorcluster)  [unwired: 7 in, 1 out]
        n75 = case shown="True" "btn test qwtb" {
          tunnel: w62 -> [w99 w113]
          tunnel: [w99 w108] -> w67
          tunnel: w66 -> [w100 w112]
          tunnel: [w100 w111] -> w64
          frame False {
          }
          frame True {
            # "test QWTB"
            n76 = call "Meas Proc QWTB Test.vi"("error in"=w113, "session in"=w112) -> ("error out"=w108:errorcluster, "ok?"=w110:bool, "session out"=w111:T2)  [unwired: 7 in]
            n77 = Unbundle By Name(w108) -> ("source"=w106:string)
            n78 = Not(x=w110) -> (.not. x?=w109:bool)
            n79 = Concatenate Strings(w106, "<tc=red><b>" ("string")) -> (w105:string)
            n80 = Select(t=w105, s=w108, f="<tc=green><b>OK") -> (s? t:f=w103:string)
            n81 = local write "qwtb status"(w109) -> ()
            n82 = call-poly "SGUI Assign String With Tags.vi"("label(s) (empty)"="qwtb stat str", "string (empty)"=w103) -> ("error out"=w101:errorcluster)  [unwired: 8 in, 1 out]
            n83 = call <vilib>:"Clear Errors.vi"("error in (no error)"=w101) -> ()  [unwired: 5 in, 2 out]
          }
        }
        n84 = Unbundle By Name(w62) -> ("status"=w98:bool)
        n85 = local write "status"(w98) -> ()
        n86 = local write "session out"(w64) -> ()
        n87 = local write "error out"(w67) -> ()
      }
      event "btn pkg ass": Value Change {
        # "Start GOLPI package manager"
        n88 = event-data() -> ()  [unwired: 1 in, 6 out]
        n89 = local read "golpi"() -> (w115:T1)
        n90 = call "GOLPI Package Assistant Panel.vi"("golpi ref"=w115) -> ("error out"=w114:errorcluster)  [unwired: 10 in]
        n91 = local write "error out"(w114) -> ()
      }
      event "btn edit startup", "btn edit exit": Value Change {
        # "startup and exit script editor"
        n92 = event-data() -> ()  [unwired: 1 in, 6 out]
        n93 = Boolean To (0,1)(Boolean="btn edit exit") -> (0, 1=w121:i16)
        n94 = Index Array(array=path[] [path "at_startup.m", path "at_exit.m"], index=w121) -> (element=w122:path)
        n95 = call "Get Root Path.vi"() -> ("root path"=w117:path)
        n96 = Build Path(base path=w117, name or relative path=path "octprog") -> (appended path=w118:path)
        n97 = Build Path(base path=w118, name or relative path=w122) -> (appended path=w120:path)
        n98 = call "Text Viewer.vi"("Path"=w120) -> ("error out"=w119:errorcluster)  [unwired: 9 in, 1 out]
        n99 = call <vilib>:"Simple Error Handler.vi"("error in (no error)"=w119) -> ()  [unwired: 4 in, 5 out]
      }
      event "btn stop": Value Change {
        # "release"
        # "close if running"
        # "get access but not start"
        # "STOP Octave"
        n100 = event-data() -> ()  [unwired: 1 in, 6 out]
        n101 = local read "golpi"() -> (w127:T1)
        n102 = call "golpi_mpc_get_access.vi"("don't query version (true)"=TRUE, "allow octave start (true)"=FALSE, "golpi session ref"=w127) -> ("error out"=w135:errorcluster, "GOLPI ref out"=w130:T111, "golpi session out"=w129:T113, "golpi session ref out (copy)"=w132:T1)  [unwired: 3 in, 2 out]
        n103 = Unbundle By Name(w129) -> ("exit command"=w128:string)
        n104 = call "golpi_mpc_close_octave.vi"("exit command (empty)"=w128, "error in"=w135, "GOLPI ref in"=w130) -> ("error out"=w134:errorcluster, "GOLPI ref out (empty)"=w133:T111)  [unwired: 6 in, 1 out]
        n105 = call "golpi_mpc_release.vi"("error in"=w134, "golpi ref or golpi session in"=w133, "golpi session ref"=w132) -> ("error out"=w131:errorcluster)  [unwired: 7 in, 1 out]
        n106 = local write "error out"(w131) -> ()
        n107 = Unbundle By Name(w131) -> ("status"=w136:bool)
        n108 = local write "status"(w136) -> ()
      }
      event "btn default": Value Change {
        # "default setup"
        n109 = event-data() -> ()  [unwired: 1 in, 6 out]
        n110 = flat-sequence {
          frame #0 {
            # "store changes"
            # "don't start octave\njust get golpi struct"
            # "This part is only to update paths that user inserted just before pushing\nbutton btn default.\nIf the path exists, it will be kept even if default values are set."
            n111 = local read "octave path"() -> (w145:path)
            n112 = local read "golpi"() -> (w142:T1)
            n113 = call "golpi_mpc_get_access.vi"("allow octave start (true)"=FALSE, "golpi session ref"=w142) -> ("error out"=w144:errorcluster, "golpi session out"=w141:T113, "golpi session ref out (copy)"=w143:T1)  [unwired: 4 in, 3 out]
            n114 = Bundle By Name(cluster=w141, "work path"=path "", "octave path"=w145) -> (w140:T113)
            n115 = call "golpi_mpc_release.vi"("error in"=w144, "golpi ref or golpi session in"=w140, "golpi session ref"=w143) -> ("error out"=w139:errorcluster)  [unwired: 7 in, 1 out]
            n116 = call <vilib>:"Clear Errors.vi"("error in (no error)"=w139) -> ()  [unwired: 5 in, 2 out]
          }
          frame #1 {
            # "set default values to structure session in"
            n117 = local read "session in"() -> (w147:T2)
            n118 = call "GOLPI Set Default Values.vi"("session in"=w147) -> ("session out"=w146:T2)  [unwired: 9 in, 1 out]
            n119 = local write "session in"(w146) -> ()
          }
          frame #2 {
            # "read out default values into GUI panel"
            n120 = local read "golpi"() -> (w153:T1)
            n121 = call "golpi_mpc_get_access.vi"("allow octave start (true)"=FALSE, "golpi session ref"=w153) -> ("error out"=w149:errorcluster, "GOLPI ref out"=w152:T111, "golpi session out"=w150:T113, "golpi session ref out (copy)"=w151:T1)  [unwired: 4 in, 2 out]
            n122 = call "golpi_mpc_release.vi"("error in"=w149, "golpi ref or golpi session in"=w152, "golpi session ref"=w151) -> ()  [unwired: 7 in, 2 out]
            n123 = Unbundle By Name(w150) -> ("start timeout [ms]"=w159:u32, "octave path"=w158:path, "console"=w157:bool, "binary"=w156:bool, "clr cache"=w155:bool, "matlab"=w154:bool)
            n124 = local write "octave path"(w158) -> ()
            n125 = local write "btn bitstream"(w156) -> ()
            n126 = local write "start timeout [ms]"(w159) -> ()
            n127 = local write "btn console"(w157) -> ()
            n128 = local write "btn clr cache"(w155) -> ()
            n129 = local write "btn matlab"(w154) -> ()
          }
        }
      }
      event "help": Value Change {
        # "Description is better than tooltip because:\n1, Description is not limited in length. Tootlip can be only 255 characters.\n2, To show the tooltip, one have to hover the mouse over the control for quite a long time."
        n130 = event-data() -> ()  [unwired: 1 in, 6 out]
        n131 = fn#1354() -> (0:w162:T114, 1:w161:bool)
        n132 = Not(x=w161) -> (.not. x?=w160:bool)
        n133 = Control Help Window(0:w162, 1:w160) -> ()
      }
    }
  }
  n134 = call "align_vi_panel.vi"() -> ()  [unwired: 11 in, 1 out]
  n135 = flat-sequence {
    tunnel: w3 -> [_]
    tunnel: w1 -> [w163]
    frame #0 {
      n136 = call "SGUI Register Controls.vi"("register mode (overwrite)"=SGUI_Assign_References_Mode."Release ID", "controls ID (empty)"=w163) -> ("error out"=w165:errorcluster)  [unwired: 15 in, 2 out]
      n137 = call <vilib>:"Clear Errors.vi"("error in (no error)"=w165) -> ()  [unwired: 5 in, 2 out]
    }
  }
  "error out" <- "error in"
  "session out" <- "session in"
